vi "phil_visualize.vi"() -> ()   [LabVIEW 2016]
uses:
  <userlib>/LevyLab/Graph Utilities/Typedefs/Histogram--slider.ctl
  subvi/ctl/Scan Info -- Cluster.ctl
  subvi/ctl/Chopper Parameters -- Cluster.ctl
  <userlib>/LevyLab/Graph Utilities/Typedefs/Histogram--Graph.ctl
  <userlib>/LevyLab/Graph Utilities/graph_utilities.lvclass
  <userlib>/LevyLab/LV to ITX/Data/Data.lvclass
  subvi/Data.S3/Data.S3.lvclass
  <userlib>/LevyLab/postgreSQL-timescaleDB/Data.PGSQL.lvclass
  <userlib>/LevyLab/Graph Utilities/graph_utilities.lvclass/graph_utilities.ctl
  <userlib>/LevyLab/LV to ITX/Data/Data.lvclass/Data.ctl
  subvi/operationQueue/fft/fft_typedef.ctl
  subvi/operationQueue/derivative/derivative_typedef.ctl
  <userlib>/_OpenG.lib/file/file.llb/File Exists - Scalar__ogtk.vi
  <userlib>/_OpenG.lib/file/file.llb/Build Path - Traditional__ogtk.vi
  <userlib>/_OpenG.lib/file/file.llb/Strip Path - Traditional__ogtk.vi
  <userlib>/_OpenG.lib/dictionary/dictionary.llb/Dictionary Update (by scalar value)__ogtk.vi
  <userlib>/LevyLab/XY Utilities/subVIs/Derivative (multiple).vi
  <userlib>/LevyLab/XY Utilities/xy_utilities.lvlib
panel:
  in  "Tab Control":enum32{"Graphs", "Page 2"}(tab)
  out "Horizontal Linecut":cluster{dbl[], dbl[]}[](graph)
  out "Vertical Linecut":cluster{dbl[], dbl[]}[](graph)
  out "Intensity Graph":dbl[][](graph)
  out "Histogram":T1
  in  "lock to bin edges":bool
  in  "# std deviations for histogram width":T2=1.4340101522842639 scale=0.0..5.0
  in  "menu select":T3(tab)
  out "Listing Indicator":bool
  out "Downloading Indicator":bool
  in  "Populate Local Tree":bool
  in  "Local Tree":string(tree)
  in  "Populate Remote Tree":bool
  in  "local bigdata directory":path=path "C:/visualization" caption="Path"
  out "Loading Indicator":bool
  out "TDMS load (ms)":u32
  in  "Remote Tree":string(tree)
  in  "path to aws credentials":path=path "C:/Users/patrick/.aws/credentials"
  in  "S3 bucket":string="levylab-data"
  out "Remote Tree load (ms)":u32
  in  "Operation Config":enum32{"derivative", "fft"}(tab)
  in  "derivative":T4={"derivative"="derivative", "Interval"=2.0, "Interval Units"=enum."Points", "Type"=enum."dy/dx vs x"}
  in  "Add Op":bool
  in  "Operations List":i32(listbox)
  in  "update":bool
  out "slicing\ntime":i32
  out "updating":bool
  in  "auto\nupdate":bool
  in  "trash can":i32(listbox)
  in  "'Z' Scale Selection (IV Y)":string(tree)
  in  "'Y' Scale Selection (IV X)":string(tree)
  out "intended sweep end":dbl
  out "actual sweep end":dbl
  in  "intended (t) end\nactual (f) end":bool
  out "scan info":T5
  in  "chopper params":T6
  out "data dimensions":i32[](array[numeric])
  out "wiring config":string[][](array[string])
  out "Notes":string
  out "Wavenames":string[](array[string])
  # "don't try to open a file that's\ncurrently downloading.."
  # "#todo: change these indicator booleans to string-based \"status\" or enum"
  # "not yet implemented"
  # "no settings"
  # "FACTS"
  # "you may find that AI7 and AI8 were not saved\ndue to an old bug in the transport stuff a while ago..\nvery unfortunate"
  # "this does virtually nothing and i am rly confused"
  # "temporary things:"
  # "Settings"
  # "4"
  # "7"
  # "10"
  # "12"
  # "14"
  # "TODO: \n-multiple file download\n-download progress indicator\n-read metadata from tdms"
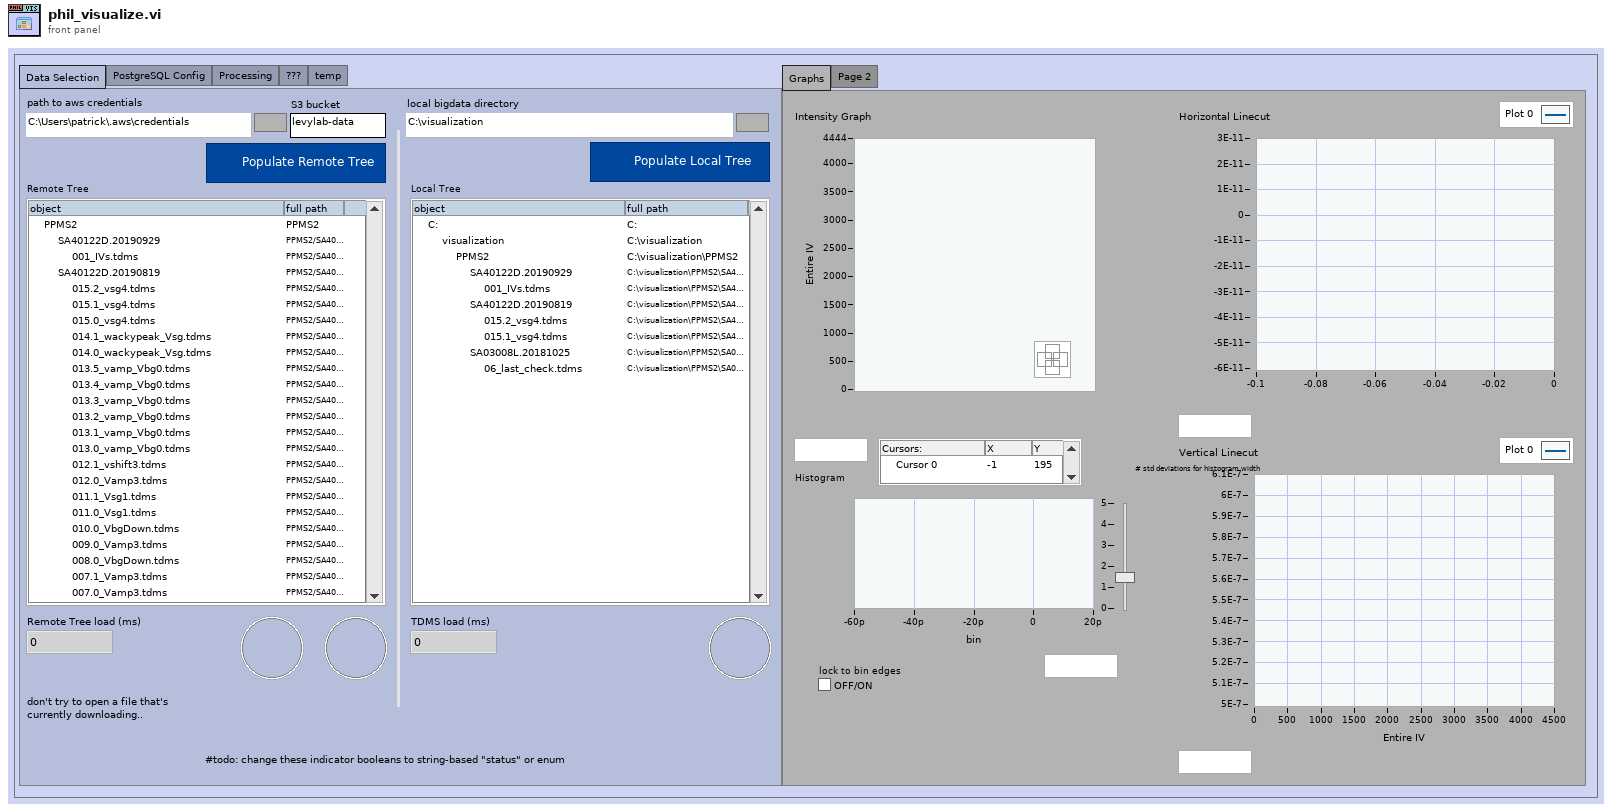
[diagram p1: front panel]
types:
  T1 = typedef "graph_utilities.lvclass/Histogram--Graph.ctl" = cluster{"X":dbl, "Y":dbl}[]
  T2 = typedef "graph_utilities.lvclass/Histogram--slider.ctl" = dbl
  T3 = enum32{"Data Selection", "PostgreSQL Config", "Processing", "???", "temp"}
  T4 = cluster{"derivative":string, "Interval":dbl, "Interval Units":enum16{"Points", "Data"}, "Type":enum16{"dy/dx vs x", "dx/dy vs y"}}
  T5 = typedef "Scan Info -- Cluster.ctl" = cluster{"scan names":string[], "starts":dbl[], "ends":dbl[], "steps":dbl[]}
  T6 = typedef "Chopper Parameters -- Cluster.ctl" = cluster{"Points to chop off the top edge":i32, "Points to chop off the bottom edge":i32, "zeroes to chop off":i32, "use auto-chopper":bool, "upper (t) or lower (f) side":bool}
  T7 = enum32{"Invalid", "Standard", "Closed", "Hidden", "Minimized", "Maximized"}
  T8 = enum32{"invalid app kind", "Development System", "Run Time System", "Student Edition", "Embedded LabVIEW", "Evaluation", "Custom"}
  T9 = typedef "fft_typedef.ctl" = cluster{"fft":string}
  T10 = typedef "derivative_typedef.ctl" = cluster{"derivative":string, "Interval":dbl, "Interval Units":enum16{"Points", "Data"}, "Type":enum16{"dy/dx vs x", "dx/dy vs y"}}
  T11 = typedef "Dictionary Object RefNum__ogtk.ctl" = refnum<k1>
  T12 = cluster{"Core":cluster{"Current VI Reference":refnum<vi>, "Close Panel on Exit?":bool}, "active XY data":cluster{"All expt data":dbl[], "All expt data":dbl[]}[], "local bigdata directory":path, "Data Save":refnum<class "Data.lvclass">, "Data.S3":refnum<class "Data.S3.lvclass">, "Data.PGSQL":refnum<class "Data.PGSQL.lvclass">, "graphs":refnum<class "graph_utilities.lvclass">[], "dictionary out":T11, "Operations List":refnum<vi>, "operations performed":string[], "Histogram Data":cluster{"X Values":dbl[], "Histogram: h(x)":i32[]}, "wavenames":string[], "data dimensions":i32[], "selected":cluster{"local path":path, "\\ remote path":string, "/ remote path":string}, "scan info":cluster{"scan names":string[], "starts":dbl[], "ends":dbl[], "steps":dbl[]}, "wiring config":string[][], "channel selection trees":cluster{"X Scale Selection":refnum<vi>, "Y Scale Selection":refnum<vi>}, "ch selection":cluster{"X Ch":string, "Y Ch":string}}
  T13 = cluster{"X Scale Selection":refnum<vi>, "Y Scale Selection":refnum<vi>}
  T14 = cluster{"scan names":string[], "starts":dbl[], "ends":dbl[], "steps":dbl[]}
  T15 = cluster{"local path":path, "\\ remote path":string, "/ remote path":string}
  T16 = cluster{"X Values":dbl[], "Histogram: h(x)":i32[]}
  T17 = cluster{"All expt data":dbl[], "All expt data":dbl[]}[]
  T18 = cluster{"Current VI Reference":refnum<vi>, "Close Panel on Exit?":bool}
  T19 = typedef "Data.lvclass/Dictionary--cluster.ctl" = cluster{"key":string, "value":variant}
  T20 = cluster{"concatenated string":string, "derivative":cluster{"derivative":string, "Interval":dbl, "Interval Units":enum16{"Points", "Data"}, "Type":enum16{"dy/dx vs x", "dx/dy vs y"}}}
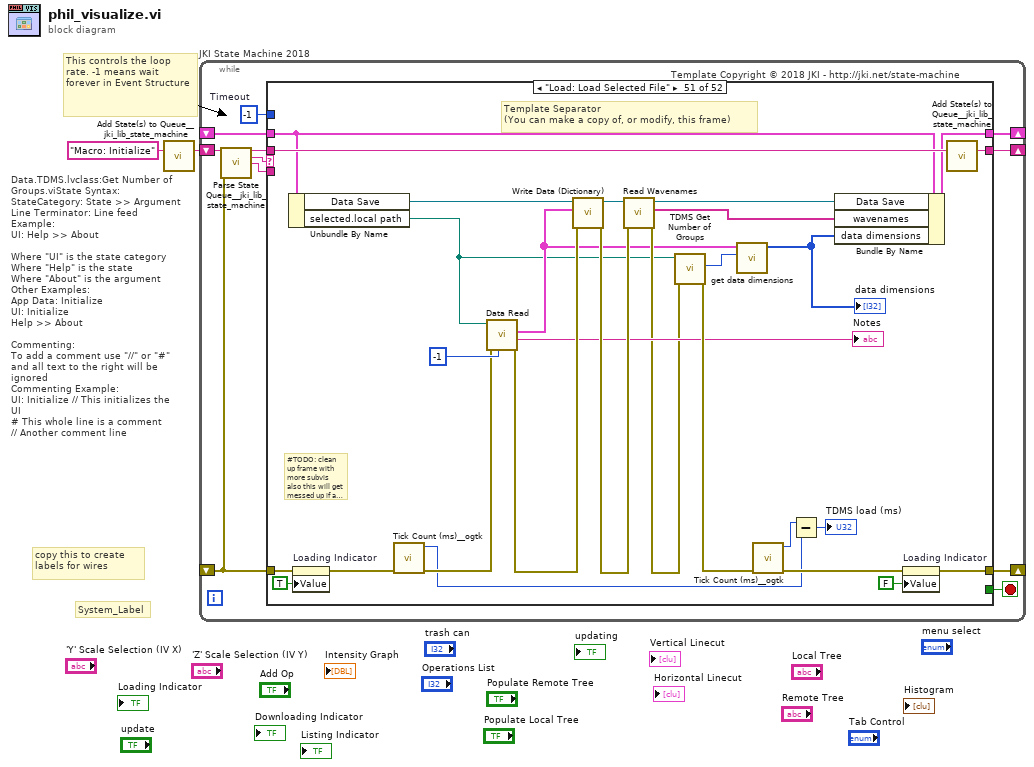
[diagram p0: block diagram]
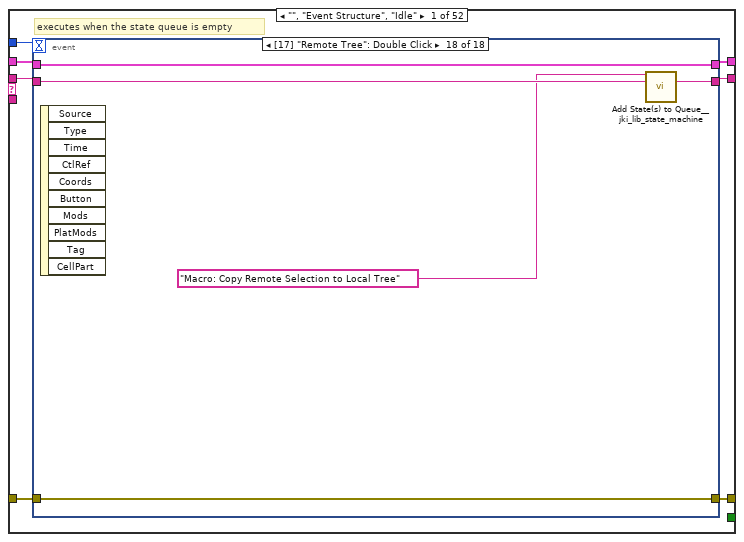
[diagram p2: hidden frame]
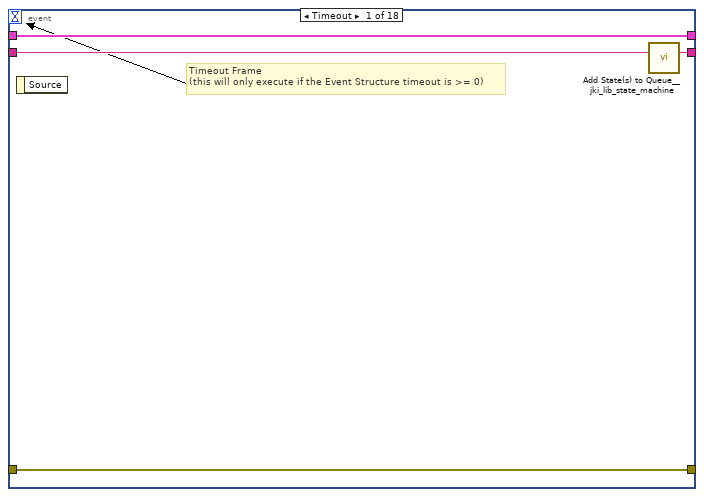
[diagram p3: hidden frame]
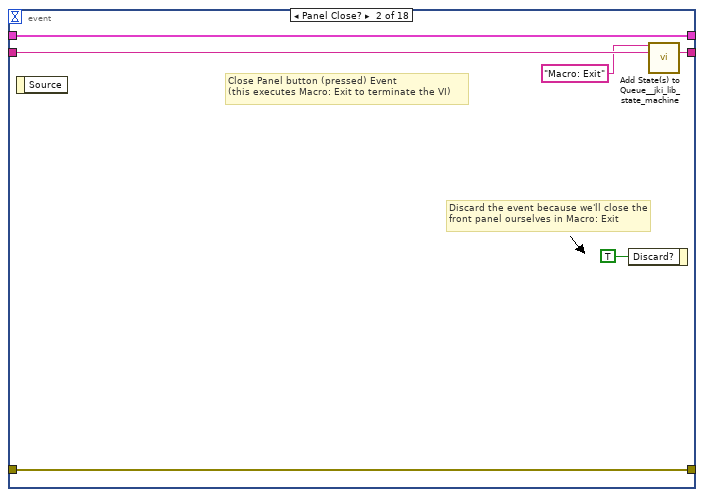
[diagram p4: hidden frame]
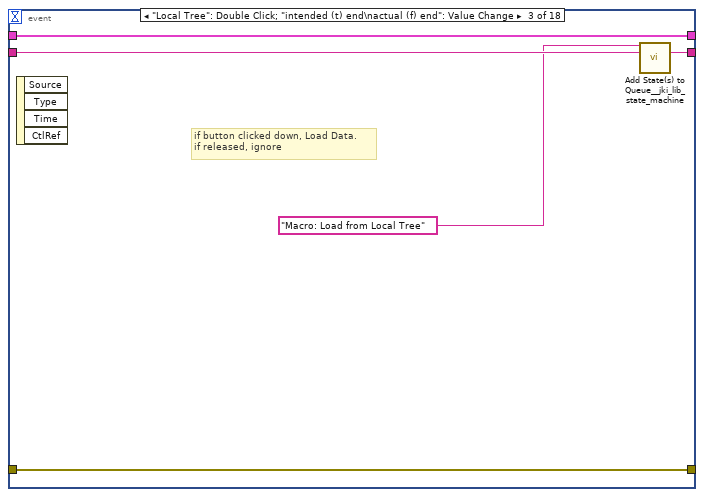
[diagram p5: hidden frame]
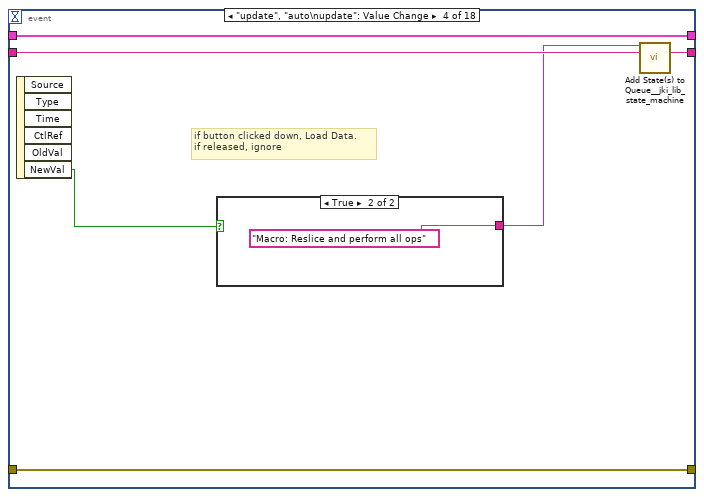
[diagram p6: hidden frame]
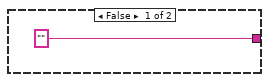
[diagram p7: hidden frame]
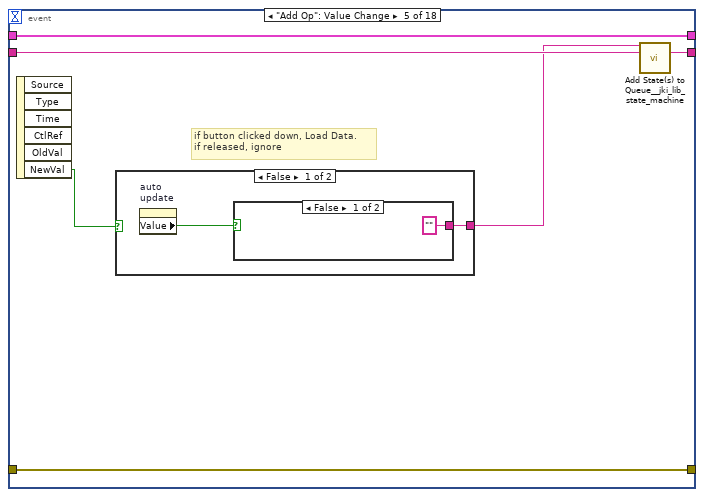
[diagram p8: hidden frame]
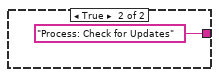
[diagram p9: hidden frame]
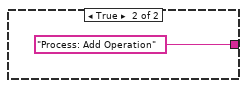
[diagram p10: hidden frame]
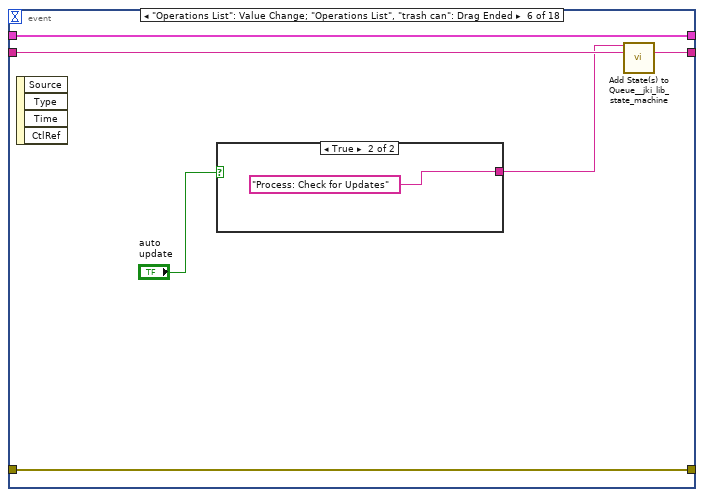
[diagram p11: hidden frame]
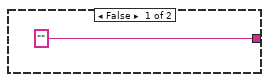
[diagram p12: hidden frame]
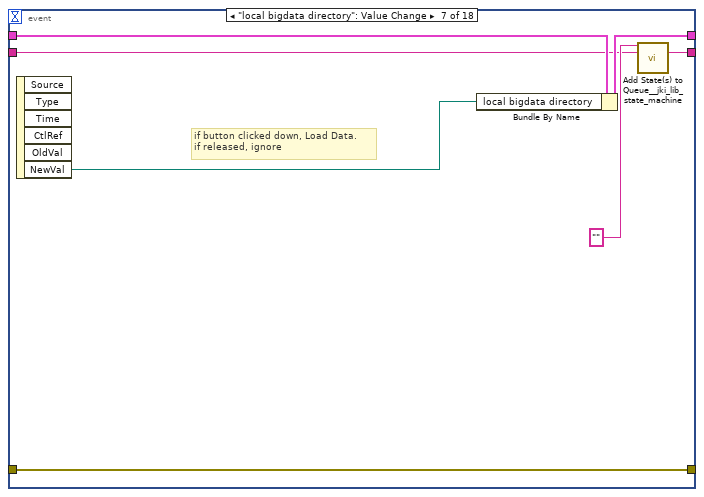
[diagram p13: hidden frame]
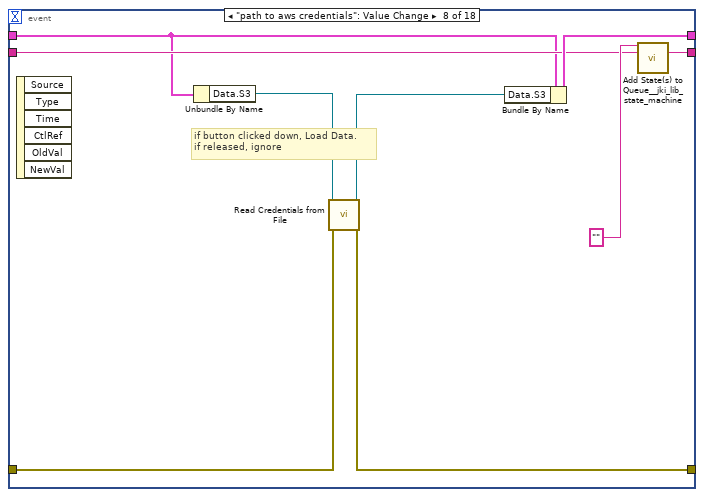
[diagram p14: hidden frame]
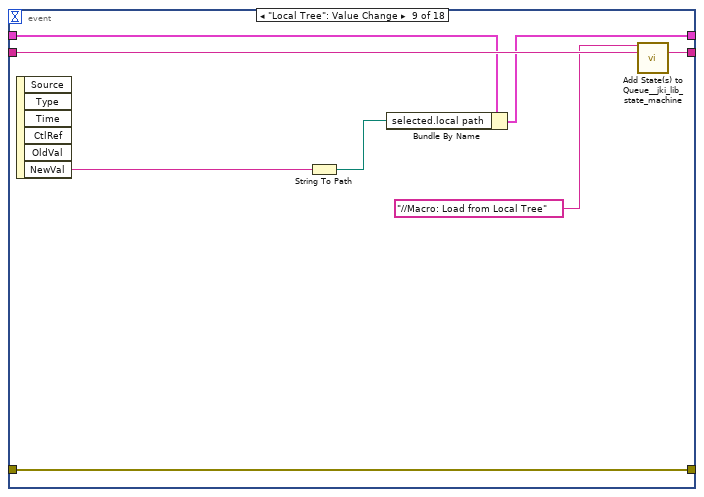
[diagram p15: hidden frame]
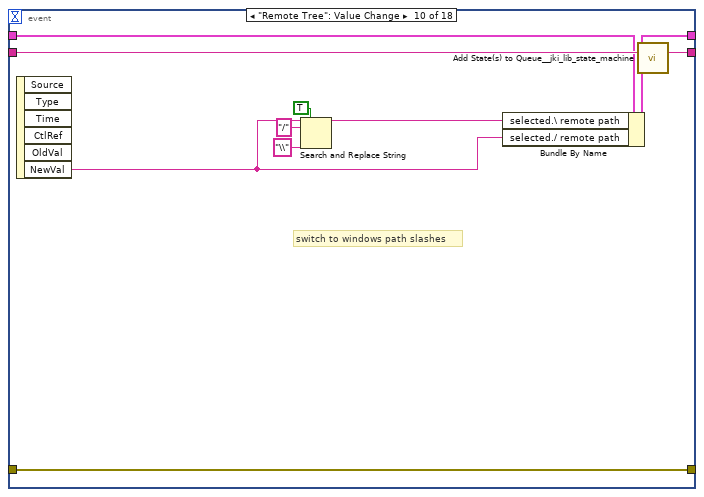
[diagram p16: hidden frame]
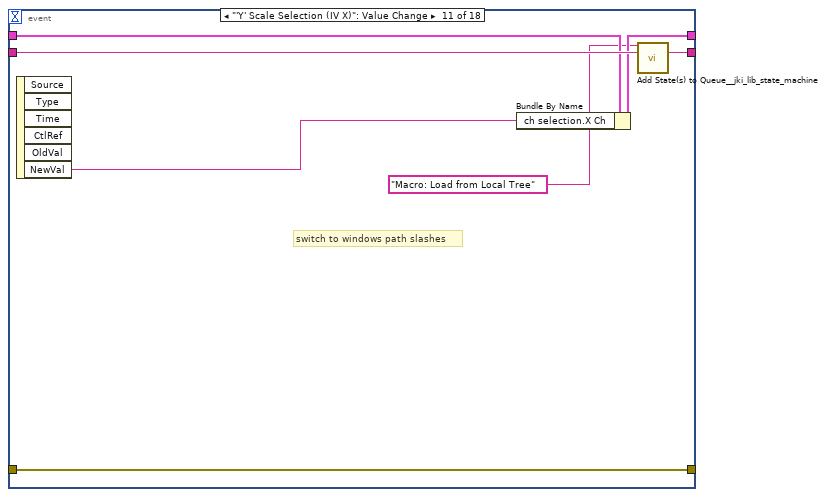
[diagram p17: hidden frame]
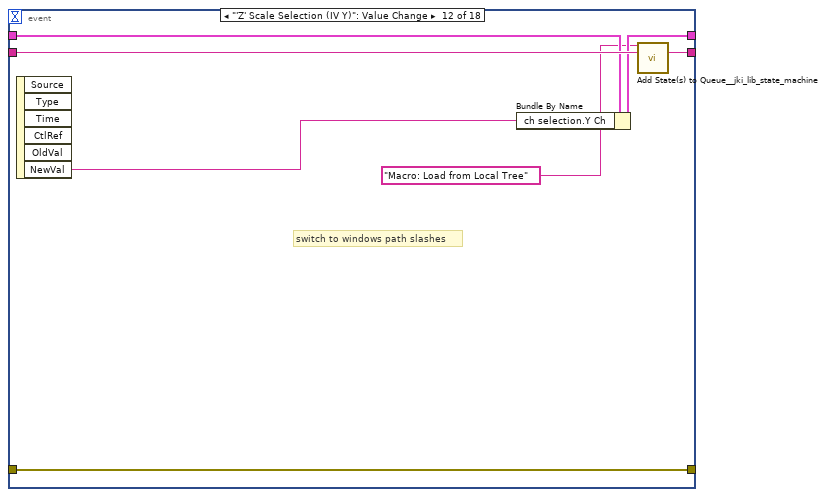
[diagram p18: hidden frame]
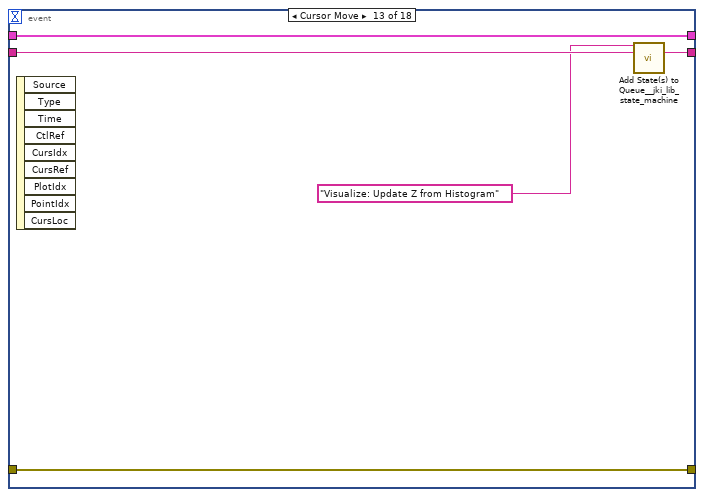
[diagram p19: hidden frame]
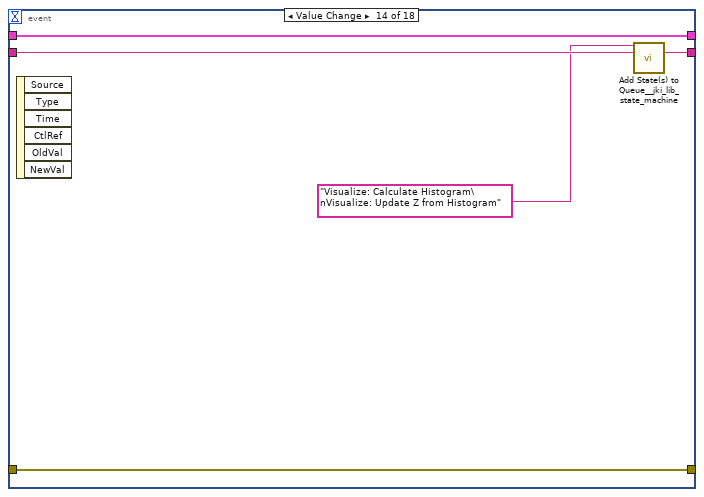
[diagram p20: hidden frame]
diagram:
  # "Data.TDMS.lvclass:Get Number of Groups.viState Syntax:\nStateCategory: State >> Argument\nLine Terminator: Line feed\nExample:\nUI: Help >> About\n\nWhere \"UI\" is the state category\nWhere \"Help\" is the state\nWhere \"About\" is the argument\nOther Examples:\nApp Data: Initialize\nUI: Initialize\nHelp >> About\n\nCommenting:\nTo add a comment use \"//\" or \"#\" and all text to the right will be ignored\nCommenting Example:\nUI: Initialize // This initializes the UI\n# This whole line is a comment\n// Another comment line"
  # "copy this to create labels for wires"
  # "This controls the loop rate. -1 means wait forever in Event Structure"
  # "System_Label"
  n1 = call <vilib>:"Add State(s) to Queue__jki_lib_state_machine.vi"("State(s) in (\"\")"="Macro: Initialize") -> ("States Out"=w2:string)  [unwired: 14 in]
  n2 = while "JKI State Machine 2018" {
    shift-right: [w6] -> _
    shift-left: _ -> [w3]
    shift-right: [w9] -> _
    shift-left: _ -> [w4]
    shift-right: [w8] -> _
    shift-left: w2 -> [w10]
    stop <- w7 stop-if-true
    w5 = -1  # Timeout
    # "Template Copyright © 2018 JKI - http://jki.net/state-machine"
    n3 = call <vilib>:"Parse State Queue__jki_lib_state_machine.vi"("State Queue"=w10, "Error In (no error)"=w4) -> ("Remaining States"=w12:string, "Current State"=w13:string, "Arguments"=w11:string)  [unwired: 11 in]
    n4 = case shown="\"Load: Load Selected File\"" w13 {
      selector: w13 -> [_ _ w151 _ _ _ _ _ _ _ _ _ _ _ _ _ _ _ _ _ _ _ _ _ _ _ _ _ _ _ _ _ _ _ _ _ _ _ _ _ _ _ _ _ _ _ _ _ _ _ _ _]
      tunnel: w12 -> [w20 w150 w155 w174 w175 w185 w189 w217 w239 w245 w249 w258 w264 w275 w344 w349 w359 w366 w371 w376 w381 w386 w391 w396 w406 w410 w414 w418 w422 w434 w452 w473 w496 w517 w529 w533 w541 w545 w549 w569 w589 w594 w620 w657 w703 w712 w732 w774 w778 w791 w823 w839]
      tunnel: w11 -> [_ _ _ _ _ _ _ _ _ _ _ _ w259 w269 _ _ _ _ _ _ _ _ _ _ _ _ _ _ _ _ _ _ _ _ _ _ _ _ _ _ _ _ _ _ _ _ _ _ _ _ _ _]
      tunnel: w3 -> [w18 w147 w153 w167 w178 w183 w186 _ w230 w240 w246 w256 w262 w271 w341 w346 w355 w363 w368 w373 w378 w383 w388 w393 w403 w407 w411 w415 w419 w430 w448 w467 w481 w505 w527 w530 w534 w542 w546 w571 w590 w600 w623 w654 w658 w708 w730 w765 w775 w789 w817 w837]
      tunnel: [w17 w148 w157 w171 errorcluster {"status"=FALSE, "code"=0, "source"=""} ("error out") w182 w187 w212 w235 w241 w247 w254 w260 w272 w342 w347 w356 w362 w367 w372 w377 w382 w387 w392 w404 w408 w412 w416 w420 w423 w435 w458 w489 w513 w523 w531 w537 w543 w547 w574 w592 w602 w624 w655 w697 w709 w728 w766 w776 w787 w819 w826] -> w9
      tunnel: w4 -> [w16 w148 w156 w171 w177 w182 w187 w213 w227 w242 w247 w255 w261 w273 w342 w347 w356 w362 w367 w372 w377 w382 w387 w392 w404 w408 w412 w416 w420 w424 w440 w462 w484 w510 w524 w531 w538 w543 w547 w575 w592 w603 w624 w655 w678 w710 w729 w767 w776 w783 w821 w835]
      tunnel: [w19 w149 w154 w173 w180 w184 w188 w216 w238 w244 w248 w257 w263 w274 w343 w348 w358 w365 w370 w375 w380 w385 w390 w395 w405 w409 w413 w417 w421 w433 w451 w472 w495 w516 w528 w532 w540 w544 w548 w569 w588 w594 w620 w656 w702 w711 w731 w773 w777 w790 w822 w838] -> w8
      tunnel: [_ _ _ _ _ TRUE _ _ _ _ _ _ _ _ _ _ _ _ _ _ _ _ _ _ _ _ _ _ _ _ _ _ _ _ _ _ _ _ _ _ _ _ _ _ _ _ _ _ _ _ _ _] -> w7
      tunnel: [w15 w147 w153 w172 w178 w183 w186 w195 w237 w240 w246 w256 w262 w271 w341 w346 w355 w363 w368 w373 w378 w383 w388 w393 w403 w407 w411 w415 w419 w429 w446 w466 w479 w505 w527 w530 w536 w542 w546 w570 w590 w600 w622 w654 w658 w708 w730 w765 w775 w789 w816 w836] -> w6
      tunnel: w5 -> [w14 _ _ _ _ _ _ _ _ _ _ _ _ _ _ _ _ _ _ _ _ _ _ _ _ _ _ _ _ _ _ _ _ _ _ _ _ _ _ _ _ _ _ _ _ _ _ _ _ _ _ _]
      frame "", "Event Structure", "Idle" {
        # "executes when the state queue is empty"
        n5 = event shown="[17] \"Remote Tree\": Double Click" {
          selector: _ -> [_ _ _ _ _ _ _ _ _ _ _ _ _ _ _ _ _ _]
          dyn-events: _ -> [_ _ _ _ _ _ _ _ _ _ _ _ _ _ _ _ _ _]
          timeout: w14 -> [_ _ _ _ _ _ _ _ _ _ _ _ _ _ _ _ _ _]
          tunnel: w20 -> [w24 w30 w32 w38 w46 w59 w64 w75 w84 w94 w101 w108 w113 w118 w122 w130 w138 w143]
          tunnel: [w23 w29 w33 w39 w47 w58 w65 w76 w85 w95 w102 w109 w112 w117 w123 w131 w139 w144] -> w19
          tunnel: w18 -> [w21 w27 w35 w41 w49 w55 w68 w74 w83 w93 w100 w107 w115 w120 w125 w133 w141 w146]
          tunnel: [w22 w28 w34 w40 w48 w60 w69 w70 w86 w96 w103 w110 w114 w119 w124 w132 w140 w145] -> w17
          tunnel: w16 -> [w22 w28 w34 w40 w48 w60 w69 w71 w86 w96 w103 w110 w114 w119 w124 w132 w140 w145]
          tunnel: [w21 w27 w35 w41 w49 w55 w67 w78 w82 w92 w99 w106 w115 w120 w125 w133 w141 w146] -> w15
          event Timeout {
            # "Timeout Frame\n(this will only execute if the Event Structure timeout is >= 0)"
            n6 = event-data() -> ()  [unwired: 1 in, 1 out]
            n7 = call <vilib>:"Add State(s) to Queue__jki_lib_state_machine.vi"("State(s) in (\"\")"=w24) -> ("States Out"=w23:string)  [unwired: 14 in]
          }
          event Panel Close? {
            # "Discard the event because we'll close the front panel ourselves in Macro: Exit"
            # "Close Panel button (pressed) Event\n(this executes Macro: Exit to terminate the VI)"
            n8 = event-data() -> ()  [unwired: 1 in, 1 out]
            n9 = event-data("Discard?"=TRUE) -> ()  [unwired: 1 in, 1 out]
            n10 = call <vilib>:"Add State(s) to Queue__jki_lib_state_machine.vi"("State(s) in Front (\"\")"="Macro: Exit", "State(s) in (\"\")"=w30) -> ("States Out"=w29:string)  [unwired: 13 in]
          }
          event "Local Tree": Double Click; "intended (t) end\nactual (f) end": Value Change {
            # "if button clicked down, Load Data.\nif released, ignore"
            n11 = event-data() -> ()  [unwired: 1 in, 4 out]
            n12 = call <vilib>:"Add State(s) to Queue__jki_lib_state_machine.vi"("State(s) in Front (\"\")"="Macro: Load from Local Tree", "State(s) in (\"\")"=w32) -> ("States Out"=w33:string)  [unwired: 13 in]
          }
          event "update", "auto\nupdate": Value Change {
            # "if button clicked down, Load Data.\nif released, ignore"
            n13 = event-data() -> ("NewVal"=w37:bool)  [unwired: 1 in, 5 out]
            n14 = case shown="True" w37 {
              tunnel: ["" "Macro: Reslice and perform all ops"] -> w36
              frame False {
              }
              frame True {
              }
            }
            n15 = call <vilib>:"Add State(s) to Queue__jki_lib_state_machine.vi"("State(s) in Front (\"\")"=w36, "State(s) in (\"\")"=w38) -> ("States Out"=w39:string)  [unwired: 13 in]
          }
          event "Add Op": Value Change {
            # "if button clicked down, Load Data.\nif released, ignore"
            n16 = event-data() -> ("NewVal"=w45:bool)  [unwired: 1 in, 5 out]
            n17 = case shown="False" w45 {
              tunnel: [w51 "Process: Add Operation"] -> w44
              frame False {
                n18 = property on="auto\nupdate" class="Bool (strict)"() -> ("Value"=w50:bool)  [unwired: 2 in, 2 out]
                n19 = case shown="False" w50 {
                  tunnel: ["" "Process: Check for Updates"] -> w51
                  frame False {
                  }
                  frame True {
                  }
                }
              }
              frame True {
              }
            }
            n20 = call <vilib>:"Add State(s) to Queue__jki_lib_state_machine.vi"("State(s) in Front (\"\")"=w44, "State(s) in (\"\")"=w46) -> ("States Out"=w47:string)  [unwired: 13 in]
          }
          event "Operations List": Value Change; "Operations List", "trash can": Drag Ended {
            n21 = event-data() -> ()  [unwired: 1 in, 4 out]
            n22 = case shown="True" "auto\nupdate" {
              tunnel: ["" "Process: Check for Updates"] -> w57
              frame False {
              }
              frame True {
              }
            }
            n23 = call <vilib>:"Add State(s) to Queue__jki_lib_state_machine.vi"("State(s) in Front (\"\")"=w57, "State(s) in (\"\")"=w59) -> ("States Out"=w58:string)  [unwired: 13 in]
          }
          event "local bigdata directory": Value Change {
            # "if button clicked down, Load Data.\nif released, ignore"
            n24 = event-data() -> ("NewVal"=w63:path)  [unwired: 1 in, 5 out]
            n25 = Bundle By Name(cluster=w68, "local bigdata directory"=w63) -> (w67:T12)
            n26 = call <vilib>:"Add State(s) to Queue__jki_lib_state_machine.vi"("State(s) in Front (\"\")"="" ("State(s) in Front (\"\")"), "State(s) in (\"\")"=w64) -> ("States Out"=w65:string)  [unwired: 13 in]
          }
          event "path to aws credentials": Value Change {
            # "if button clicked down, Load Data.\nif released, ignore"
            n27 = event-data() -> ()  [unwired: 1 in, 6 out]
            n28 = Unbundle By Name(w74) -> ("Data.S3"=w73:refnum<class "Data.S3.lvclass">)
            n29 = call "Read Credentials from File.vi"("error in (no error)"=w71, "Data.S3"=w73) -> ("error out"=w70:errorcluster, "Data.S3 out"=w72:refnum<class "Data.S3.lvclass">)  [unwired: 8 in]
            n30 = Bundle By Name(cluster=w74, "Data.S3"=w72) -> (w78:T12)
            n31 = call <vilib>:"Add State(s) to Queue__jki_lib_state_machine.vi"("State(s) in Front (\"\")"="" ("State(s) in Front (\"\")"), "State(s) in (\"\")"=w75) -> ("States Out"=w76:string)  [unwired: 13 in]
          }
          event "Local Tree": Value Change {
            n32 = event-data() -> ("NewVal"=w80:string)  [unwired: 1 in, 5 out]
            n33 = String To Path(string=w80) -> (path=w81:path)
            n34 = Bundle By Name(cluster=w83, "selected.local path"=w81) -> (w82:T12)
            n35 = call <vilib>:"Add State(s) to Queue__jki_lib_state_machine.vi"("State(s) in Front (\"\")"="//Macro: Load from Local Tree", "State(s) in (\"\")"=w84) -> ("States Out"=w85:string)  [unwired: 13 in]
          }
          event "Remote Tree": Value Change {
            # "switch to windows path slashes"
            n36 = event-data() -> ("NewVal"=w88:string)  [unwired: 1 in, 5 out]
            n37 = Search and Replace String(replace all?=TRUE ("replace all? (F)"), input string=w88, search string="/", replace string="\\" ("replace string (\"\")")) -> (result string=w89:string)  [unwired: 4 in, 3 out]
            n38 = Bundle By Name(cluster=w93, "selected.\\ remote path"=w89, "selected./ remote path"=w88) -> (w92:T12)
            n39 = call <vilib>:"Add State(s) to Queue__jki_lib_state_machine.vi"("State(s) in (\"\")"=w94) -> ("States Out"=w95:string)  [unwired: 14 in]
          }
          event "'Y' Scale Selection (IV X)": Value Change {
            # "switch to windows path slashes"
            n40 = event-data() -> ("NewVal"=w98:string)  [unwired: 1 in, 5 out]
            n41 = Bundle By Name(cluster=w100, "ch selection.X Ch"=w98) -> (w99:T12)
            n42 = call <vilib>:"Add State(s) to Queue__jki_lib_state_machine.vi"("State(s) in Front (\"\")"="Macro: Load from Local Tree", "State(s) in (\"\")"=w101) -> ("States Out"=w102:string)  [unwired: 13 in]
          }
          event "'Z' Scale Selection (IV Y)": Value Change {
            # "switch to windows path slashes"
            n43 = event-data() -> ("NewVal"=w105:string)  [unwired: 1 in, 5 out]
            n44 = Bundle By Name(cluster=w107, "ch selection.Y Ch"=w105) -> (w106:T12)
            n45 = call <vilib>:"Add State(s) to Queue__jki_lib_state_machine.vi"("State(s) in Front (\"\")"="Macro: Load from Local Tree", "State(s) in (\"\")"=w108) -> ("States Out"=w109:string)  [unwired: 13 in]
          }
          event Cursor Move {
            n46 = event-data() -> ()  [unwired: 1 in, 9 out]
            n47 = call <vilib>:"Add State(s) to Queue__jki_lib_state_machine.vi"("State(s) in Front (\"\")"="Visualize: Update Z from Histogram" ("State(s) in Front (\"\")"), "State(s) in (\"\")"=w113) -> ("States Out"=w112:string)  [unwired: 13 in]
          }
          event Value Change {
            n48 = event-data() -> ()  [unwired: 1 in, 6 out]
            n49 = call <vilib>:"Add State(s) to Queue__jki_lib_state_machine.vi"("State(s) in Front (\"\")"="Visualize: Calculate Histogram\nVisualize: Update Z from Histogram" ("State(s) in Front (\"\")"), "State(s) in (\"\")"=w118) -> ("States Out"=w117:string)  [unwired: 13 in]
          }
          event "Intensity Graph": Cursor Move {
            n50 = event-data() -> ()  [unwired: 1 in, 9 out]
            n51 = call <vilib>:"Add State(s) to Queue__jki_lib_state_machine.vi"("State(s) in Front (\"\")"="Visualize: Line Cuts" ("State(s) in Front (\"\")"), "State(s) in (\"\")"=w122) -> ("States Out"=w123:string)  [unwired: 13 in]
          }
          event "Populate Remote Tree": Value Change {
            n52 = event-data() -> ("NewVal"=w129:bool)  [unwired: 1 in, 5 out]
            n53 = Select(t="Macro: Populate Remote Tree" ("State(s) in Front (\"\")"), s=w129, f="") -> (s? t:f=w126:string)
            n54 = call <vilib>:"Add State(s) to Queue__jki_lib_state_machine.vi"("State(s) in Front (\"\")"=w126, "State(s) in (\"\")"=w130) -> ("States Out"=w131:string)  [unwired: 13 in]
          }
          event "Populate Local Tree": Value Change {
            n55 = event-data() -> ("NewVal"=w137:bool)  [unwired: 1 in, 5 out]
            n56 = Select(t="Macro: Populate Local Tree" ("State(s) in Front (\"\")"), s=w137, f="") -> (s? t:f=w134:string)
            n57 = call <vilib>:"Add State(s) to Queue__jki_lib_state_machine.vi"("State(s) in Front (\"\")"=w134, "State(s) in (\"\")"=w138) -> ("States Out"=w139:string)  [unwired: 13 in]
          }
          event "Remote Tree": Double Click {
            n58 = event-data() -> ()  [unwired: 1 in, 10 out]
            n59 = call <vilib>:"Add State(s) to Queue__jki_lib_state_machine.vi"("State(s) in Front (\"\")"="Macro: Copy Remote Selection to Local Tree" ("State(s) in Front (\"\")"), "State(s) in (\"\")"=w143) -> ("States Out"=w144:string)  [unwired: 13 in]
          }
        }
      }
      frame "---------- Core ----------" {
        # "Do not put any code in this frame.\n(it is a separator no-op)"
        n60 = call <vilib>:"Add State(s) to Queue__jki_lib_state_machine.vi"("State(s) in (\"\")"=w150) -> ("States Out"=w149:string)  [unwired: 14 in]
      }
      frame Default {
        w160 = 42 items=["No error", "Argument error", "Memory is full", "Out of zone", "End of file", "File already open", "Generic file I/O error", "File not found", "File permission error", "Disk is full", "Duplicate path", "Too many files open", "System feature not enabled", "Resource file not found", "Cannot add resource", "Resource not found", "Image not found", "Image memory error", "Pen does not exist", "Config type invalid", "Config token not found", "Config parse error", "Config memory error", "Bad external code format", "Bad external code offset", "External code not present", "Null window", "Destroy window error", "Null menu", "Print aborted", "Bad print record", "Print driver error", "Windows error during printing", "Memory error during printing", "Print dialog error", "Generic print error", "Invalid device refnum", "Device not found", "Device parameter error", "Device unit error", "Cannot open device", "Device call aborted", "Generic error", "Cancelled by user", "Object ID too low", "Object ID too high", "Object not in heap", "Unknown heap", "Unknown object (invalid DefProc)", "Unknown object (DefProc not in table)", "Message out of range", "Invalid (null) method", "Unknown message", "Manager call not supported", "Bad address", "Network operation in progress", "Network operation timed out", "Connection is busy", "Network attribute not supported", "Network error", "Address in use", "System out of memory", "Connection aborted", "Connection refused", "Not connected", "Already connected", "Connection closed", "Initialization error (interapplication manager)", "Bad occurrence", "Wait on unbound occurrence handler", "Occurrence queue overflow", "Datalog type conflict", "Unused", "Unrecognized type (interapplication manager)", "Memory corrupt", "Failed to make temporary DLL", "Old CIN version", "Drag socket not found", "Failed to load drop-object", "Failed to register OLE object", "Failed to release OLE object", "Format specifier type mismatch", "Unknown format specifier", "Too few format specifiers", "Too many format specifiers", "Scan failed", "Newer CIN version", "Error converting to variant", "Runtime menu error", "Password tampered", "Variant attribute not found", "Incompatible variant data type", "Event data is not available", "Event Store is not present", "Occurrence is not found", "Event Queue is not created", "Event info is not available", "Refnum passed is NULL", "Error retrieving Class GUID", "Error retrieving CoClass GUID", "Error retrieving TypeLib GUID.", "Bad built application magic bytes.", "Specific driver is different from the specific driver associated with the Logical Name.", "There is no session opened to the class driver.", "Max Error", "MAX - Error with config objects", "MAX - Error loading configuration", "MAX - Group not supported"]
        # "Current State"
        # "Do not delete, rename, or modify this frame.\n(this is used to capture unhandled states and typos)"
        # "Handle mistyped state name (developer tool)"
        n61 = Format Into String(format string="Software Exception: Unhandled State \"%s\"." ("message"), error in=w156, w151) -> (resulting string=w159:string, error out=w158:errorcluster)  [unwired: 1 in]
        n62 = call <vilib>:"Error Cluster From Error Code.vi"("show call chain? (False)"=TRUE, "error in (no error)"=w158, "error message (\"\")"=w159, "error code (0)"=w160) -> ("error out"=w157:errorcluster)  [unwired: 5 in]
        n63 = call <vilib>:"Add State(s) to Queue__jki_lib_state_machine.vi"("State(s) in (\"\")"=w155) -> ("States Out"=w154:string)  [unwired: 14 in]
      }
      frame "Initialize Core Data" {
        # "Do not delete, rename, or modify this frame.\n(this is used to determine panel behavior on exit)"
        # "originally closed?"
        # "exe?"
        # "If panel starts closed or is an EXE, then close it when we exit"
        n64 = property class="VI"() -> ("FP.State"=w164:T7)  [unwired: 2 in, 2 out]
        n65 = property class="App"() -> ("App.Kind"=w170:T8)  [unwired: 2 in, 2 out]
        n66 = control-ref of="Current VI Reference"() -> (w165:refnum<vi>)
        n67 = Equal?(x=w164, y=T7."Closed" ("Front Panel Window:State")) -> (x = y?=w162:bool)
        n68 = Equal?(x=w170, y=T8."Run Time System" ("Application:Kind")) -> (x = y?=w168:bool)
        n69 = Or(x=w162, y=w168) -> (x .or. y?=w166:bool)
        n70 = Bundle By Name(cluster=w167, "Core.Current VI Reference"=w165, "Core.Close Panel on Exit?"=w166) -> (w172:T12)
        n71 = call <vilib>:"Add State(s) to Queue__jki_lib_state_machine.vi"("State(s) in (\"\")"=w174) -> ("States Out"=w173:string)  [unwired: 14 in]
      }
      frame "Error Handler" {
        # "Unhandled Error -- Display it"
        # "Handle any errors here.\nYou can also output any states to clean-up after errors occur"
        # "Clear error"
        n72 = call <vilib>:"General Error Handler.vi"("error in (no error)"=w177) -> ()  [unwired: 10 in, 5 out]
        n73 = call <vilib>:"Add State(s) to Queue__jki_lib_state_machine.vi"("State(s) in Front (\"\")"="/* Post Error States", "State(s) in (\"\")"=w175) -> ("States Out"=w180:string)  [unwired: 13 in]
      }
      frame "Exit" {
        # "Do not put any code in this frame.\n(No errors that occur here will be handled.)"
        n74 = call <vilib>:"Add State(s) to Queue__jki_lib_state_machine.vi"("State(s) in (\"\")"=w185) -> ("States Out"=w184:string)  [unwired: 14 in]
      }
      frame "---------- Data ----------" {
        # "Do not put any code in this frame.\n(It is a separator no-op. You can make a copy of this frame to create a new Data frame)"
        n75 = call <vilib>:"Add State(s) to Queue__jki_lib_state_machine.vi"("State(s) in (\"\")"=w189) -> ("States Out"=w188:string)  [unwired: 14 in]
      }
      frame "Data: Initialize" {
        w191 = refnum<class "Data.PGSQL.lvclass"> refnum  # Data.PGSQL
        w196 = cluster{"X Ch":string, "Y Ch":string} {"X Ch"="AO3", "Y Ch"="AI4"}  # ch selection
        w197 = T13 {"X Scale Selection"=refnum, "Y Scale Selection"=refnum}  # channel selection trees
        w201 = string[][] []  # wiring config
        w202 = T14 {"scan names"=["DSA_Vsg1", "OFF", "OFF", "OFF"], "starts"=[-1.0, 0.0, 0.2, 0.0], "ends"=[1.0, 0.2, 0.3, 0.5], "steps"=[0.005, 0.001, 0.025, 0.01]}  # scan info
        w203 = T15 {"local path"=path "", "\\ remote path"="", "/ remote path"=""}  # selected
        w204 = i32[] []  # data dimensions
        w192 = refnum<class "Data.S3.lvclass"> refnum  # Data.S3
        w205 = string[] []  # wavenames
        w194 = refnum<class "Data.lvclass"> refnum  # Data Save
        w206 = T16 {"X Values"=[], "Histogram: h(x)"=[]}  # Histogram Data
        w207 = string[] []  # operations performed
        w209 = T17 []  # active XY data
        w208 = string[] [] ("Strings []")
        w193 = refnum<class "graph_utilities.lvclass">[] []  # graphs
        w215 = T18 {"Current VI Reference"=refnum, "Close Panel on Exit?"=FALSE}  # Core
        # "# groups in tdms\n    (i.e. # original itx files)\n# channels (time, AIN, AON,\n# points per channel\n    (except the channels\n     that only store 1)"
        # "do not delete - used by framework"
        # "Data names and types of shift register data are defined by this bundle."
        # "Initialize the shift-register data, here.\n(data names are defined by what you wire into the bundle function)"
        n76 = call <userlib>:"Dictionary Create__ogtk.vi"("error in (no error)"=w213) -> ("error out"=w212:errorcluster, "dictionary out"=w214:T11)  [unwired: 9 in]
        n77 = control-ref of="Operations List"() -> (w210:refnum<vi>)
        n78 = property on="trash can" class="LstBox (strict)"("Item Names"=w208) -> ()  [unwired: 2 in, 2 out]
        n79 = property class="LstBox (strict)"(reference=w210, "Item Names"=w208) -> (reference out=w211:refnum<vi>)  [unwired: 1 in, 1 out]
        n80 = control-ref of="'Y' Scale Selection (IV X)"() -> (w200:refnum<vi>)
        n81 = control-ref of="'Z' Scale Selection (IV Y)"() -> (w199:refnum<vi>)
        n82 = Bundle(cluster=w197, "X Scale Selection"=w200, "Y Scale Selection"=w199) -> (w198:T13)
        n83 = Bundle("Core"=w215, "active XY data"=w209, "local bigdata directory"="local bigdata directory", "Data Save"=w194, "Data.S3"=w192, "Data.PGSQL"=w191, "graphs"=w193, "dictionary out"=w214, "Operations List"=w211, "operations performed"=w207, "Histogram Data"=w206, "wavenames"=w205, "data dimensions"=w204, "selected"=w203, "scan info"=w202, "wiring config"=w201, "channel selection trees"=w198, "ch selection"=w196) -> (w195:T12)  [unwired: 1 in]
        n84 = call <vilib>:"Add State(s) to Queue__jki_lib_state_machine.vi"("State(s) in (\"\")"=w217) -> ("States Out"=w216:string)  [unwired: 14 in]
      }
      frame "Data: Initialize Graph References" {
        # "#todo\nmove elsewhere"
        # "clear graph"
        n85 = invoke on="Remote Tree" class="Tree (strict)" method="Edit Tree Items.Delete"(error in=w227) -> (error out=w226:errorcluster)  [unwired: 4 in, 4 out]
        n86 = control-ref of="Intensity Graph"() -> (w218:refnum<vi>)
        n87 = property class="IntGraph (strict)"(reference=w218, "Value"=dbl[][] []) -> (reference out=w228:refnum<vi>)  [unwired: 1 in, 1 out]
        n88 = invoke on="Local Tree" class="Tree (strict)" method="Edit Tree Items.Delete"(error in=w226) -> (error out=w225:errorcluster)  [unwired: 4 in, 4 out]
        n89 = control-ref of="Histogram"() -> (w220:refnum<vi>)
        n90 = control-ref of="Vertical Linecut"() -> (w232:refnum<vi>)
        n91 = control-ref of="Horizontal Linecut"() -> (w233:refnum<vi>)
        n92 = call <userlib>:"Write Intensity Graph ref.vi"("error in (no error)"=w225, "Intensity Graph (Control)"=w228, "Intensity Graph"=w228) -> ("error out"=w222:errorcluster, "graph_utilities out"=w224:refnum<class "graph_utilities.lvclass">)  [unwired: 7 in]
        n93 = call <userlib>:"Write XY Graph ref.vi"("error in (no error)"=w222, "XY Graph"=w220, "graph_utilities in"=w224) -> ("error out"=w221:errorcluster, "graph_utilities out"=w223:refnum<class "graph_utilities.lvclass">)  [unwired: 7 in]
        n94 = call <userlib>:"Write XY Graph ref.vi"("error in (no error)"=w221, "XY Graph"=w232, "graph_utilities in"=w224) -> ("error out"=w236:errorcluster, "graph_utilities out"=w231:refnum<class "graph_utilities.lvclass">)  [unwired: 7 in]
        n95 = call <userlib>:"Write XY Graph ref.vi"("error in (no error)"=w236, "XY Graph"=w233, "graph_utilities in"=w224) -> ("error out"=w235:errorcluster, "graph_utilities out"=w234:refnum<class "graph_utilities.lvclass">)  [unwired: 7 in]
        n96 = Build Array(w223, w231, w234) -> (w219:refnum<class "graph_utilities.lvclass">[])
        n97 = Bundle By Name(cluster=w230, "graphs"=w219) -> (w237:T12)
        n98 = call <vilib>:"Add State(s) to Queue__jki_lib_state_machine.vi"("State(s) in (\"\")"=w239) -> ("States Out"=w238:string)  [unwired: 14 in]
      }
      frame "Data: Cleanup" {
        # "Cleanup any data and references, here.\n(this is called automatically, by the Macro: Exit)"
        n99 = Unbundle By Name(w240) -> ("Core.Current VI Reference"=w243:refnum<vi>)
        n100 = Close Reference(reference=w243, error in (no error)=w242) -> (error out=w241:errorcluster)
        n101 = call <vilib>:"Add State(s) to Queue__jki_lib_state_machine.vi"("State(s) in (\"\")"=w245) -> ("States Out"=w244:string)  [unwired: 14 in]
      }
      frame "---------- UI ----------" {
        # "Do not put any code in this frame.\n(It is a separator no-op. You can make a copy of this frame to create a new UI frame)"
        n102 = call <vilib>:"Add State(s) to Queue__jki_lib_state_machine.vi"("State(s) in (\"\")"=w249) -> ("States Out"=w248:string)  [unwired: 14 in]
      }
      frame "UI: Initialize" {
        w250 = FALSE ("Loading Indicator")
        # "Initialize the User Interface, here.\n(this is called automatically, by the Macro: Init)"
        n103 = call <userlib>:"Fit VI window to Largest Dec__ogtk.vi"("error in (no error)"=w255, "border spacing (2 px)"=-2) -> ("error out"=w254:errorcluster)  [unwired: 4 in, 1 out]
        n104 = local write "Loading Indicator"(w250) -> ()
        n105 = local write "Downloading Indicator"(w250) -> ()
        n106 = local write "Remote Tree load (ms)"(u32 0 ("Remote Tree load (ms)")) -> ()
        n107 = local write "TDMS load (ms)"(u32 0 ("TDMS load (ms)")) -> ()
        n108 = local write "Listing Indicator"(w250) -> ()
        n109 = call <vilib>:"Add State(s) to Queue__jki_lib_state_machine.vi"("State(s) in (\"\")"=w258) -> ("States Out"=w257:string)  [unwired: 14 in]
      }
      frame "UI: Cursor Set" {
        # "Argument"
        # "Set and Unset Cursor Busy.\n(Usage: \"UI: Cursor Set >> Busy|Idle\")"
        n110 = case shown="\"Idle\", Default" w259 {
          tunnel: w261 -> [w266 w268]
          tunnel: [w265 w267] -> w260
          frame "Idle", Default {
            n111 = call <vilib>:"Unset Busy.vi"("error in (no error)"=w266) -> ("error out"=w265:errorcluster)  [unwired: 10 in]
          }
          frame "Busy" {
            n112 = call <vilib>:"Set Busy.vi"("error in (no error)"=w268) -> ("error out"=w267:errorcluster)  [unwired: 9 in, 1 out]
          }
        }
        n113 = call <vilib>:"Add State(s) to Queue__jki_lib_state_machine.vi"("State(s) in (\"\")"=w264) -> ("States Out"=w263:string)  [unwired: 14 in]
      }
      frame "UI: Front Panel State" {
        # "Argument"
        # "Set Front Panel Open or Closed\n(Usage: \"UI: Front Panel State >> Open|Close\")"
        n114 = Unbundle By Name(w271) -> ("Core.Current VI Reference"=w270:refnum<vi>)
        n115 = case shown="\"Minimize\", \"Minimized\"" w269 {
          tunnel: w273 -> [w281 w296 w307 w320 w333]
          tunnel: [w283 w297 w309 w322 w335] -> w272
          tunnel: w270 -> [w282 w294 w308 w321 w334]
          frame "Open", "Standard", Default {
            w276 = T7."Standard" ("State")
            n116 = property class="VI"(reference=w282, error in=w281) -> (reference out=w279:refnum<vi>, error out=w280:errorcluster, "FP.State"=w278:T7)
            n117 = Not Equal?(x=w278, y=w276) -> (x != y?=w277:bool)
            n118 = case shown="True" w277 {
              tunnel: [w287 w289] -> w283
              tunnel: w280 -> [w286 w289]
              tunnel: w279 -> [w285 _]
              tunnel: w276 -> [w284 _]
              frame True {
                n119 = invoke class="VI" method="FP.Open"(reference=w285, error in=w286, "Activate"=TRUE, "State"=w284) -> (error out=w287:errorcluster)  [unwired: 1 in, 4 out]
              }
              frame False {
              }
            }
          }
          frame "Close", "Closed" {
            n120 = property class="VI"(reference=w294, error in=w296) -> (reference out=w293:refnum<vi>, error out=w295:errorcluster, "FP.State"=w291:T7)
            n121 = Not Equal?(x=w291, y=T7."Closed" ("Front Panel Window:State")) -> (x != y?=w290:bool)
            n122 = case shown="True" w290 {
              tunnel: [w298 w301] -> w297
              tunnel: w295 -> [w298 w300]
              tunnel: w293 -> [_ w299]
              frame False {
              }
              frame True {
                n123 = invoke class="VI" method="FP.Close"(reference=w299, error in=w300) -> (error out=w301:errorcluster)  [unwired: 1 in, 2 out]
              }
            }
          }
          frame "Hidden", "Hide" {
            w302 = T7."Hidden" ("State")
            n124 = property class="VI"(reference=w308, error in=w307) -> (reference out=w305:refnum<vi>, error out=w306:errorcluster, "FP.State"=w304:T7)
            n125 = Not Equal?(x=w304, y=w302) -> (x != y?=w303:bool)
            n126 = case shown="True" w303 {
              tunnel: [w313 w314] -> w309
              tunnel: w306 -> [w312 w314]
              tunnel: w305 -> [w311 _]
              tunnel: w302 -> [w310 _]
              frame True {
                n127 = invoke class="VI" method="FP.Open"(reference=w311, error in=w312, "State"=w310) -> (error out=w313:errorcluster)  [unwired: 2 in, 4 out]
              }
              frame False {
              }
            }
          }
          frame "Minimize", "Minimized" {
            w315 = T7."Minimized" ("State")
            n128 = property class="VI"(reference=w321, error in=w320) -> (reference out=w318:refnum<vi>, error out=w319:errorcluster, "FP.State"=w317:T7)
            n129 = Not Equal?(x=w317, y=w315) -> (x != y?=w316:bool)
            n130 = case shown="True" w316 {
              tunnel: [w326 w327] -> w322
              tunnel: w319 -> [w325 w327]
              tunnel: w318 -> [w324 _]
              tunnel: w315 -> [w323 _]
              frame True {
                n131 = invoke class="VI" method="FP.Open"(reference=w324, error in=w325, "State"=w323) -> (error out=w326:errorcluster)  [unwired: 2 in, 4 out]
              }
              frame False {
              }
            }
          }
          frame "Maximize", "Maximized" {
            w328 = T7."Maximized" ("State")
            n132 = property class="VI"(reference=w334, error in=w333) -> (reference out=w331:refnum<vi>, error out=w332:errorcluster, "FP.State"=w330:T7)
            n133 = Not Equal?(x=w330, y=w328) -> (x != y?=w329:bool)
            n134 = case shown="True" w329 {
              tunnel: [w339 w340] -> w335
              tunnel: w332 -> [w338 w340]
              tunnel: w331 -> [w337 _]
              tunnel: w328 -> [w336 _]
              frame True {
                n135 = invoke class="VI" method="FP.Open"(reference=w337, error in=w338, "State"=w336) -> (error out=w339:errorcluster)  [unwired: 2 in, 4 out]
              }
              frame False {
              }
            }
          }
        }
        n136 = call <vilib>:"Add State(s) to Queue__jki_lib_state_machine.vi"("State(s) in (\"\")"=w275) -> ("States Out"=w274:string)  [unwired: 14 in]
      }
      frame "---------- Macro ----------" {
        # "Do not put any code in this frame.\n(It is a separator no-op. You can make a copy of this frame to create a new Macro frame)"
        n137 = call <vilib>:"Add State(s) to Queue__jki_lib_state_machine.vi"("State(s) in (\"\")"=w344) -> ("States Out"=w343:string)  [unwired: 14 in]
      }
      frame "Macro: Initialize" {
        # "Initialization Macro\n(This is called once, when the VI starts)"
        n138 = call <vilib>:"Add State(s) to Queue__jki_lib_state_machine.vi"("State(s) in Front (\"\")"="Data: Initialize\nData: Initialize Graph References\nInitialize Core Data\nUI: Initialize\nUI: Front Panel State >> Open", "State(s) in (\"\")"=w349) -> ("States Out"=w348:string)  [unwired: 13 in]
      }
      frame "Macro: Load from Local Tree" {
        # "Initialization Macro\n(This is called once, when the VI starts)"
        n139 = Unbundle By Name(w355) -> ("selected.local path"=w354:path)
        n140 = call-poly <userlib>:"File Exists__ogtk.vi"("file path"=w354) -> ("is directory"=w353:bool, "exists"=w351:bool)  [unwired: 6 in]
        n141 = Not(x=w353) -> (.not. x?=w352:bool)
        n142 = And(x=w352, y=w351) -> (x .and. y?=w350:bool)
        n143 = case shown="True" w350 {
          tunnel: [" " "UI: Cursor Set >> Busy\nLoad: Load Selected File\nLoad: Load Metadata\nProcess: Slice to XY data\nMacro: Visualize\nUI: Cursor Set >> Idle"] -> w357
          frame False {
            n144 = call "Display Message to User2"() -> ()  [unwired: 10 in, 2 out]
          }
          frame True {
          }
        }
        n145 = call <vilib>:"Add State(s) to Queue__jki_lib_state_machine.vi"("State(s) in Front (\"\")"=w357, "State(s) in (\"\")"=w359) -> ("States Out"=w358:string)  [unwired: 13 in]
      }
      frame "Macro: Populate Remote Tree" {
        # "#TODO: should make sure AWS is configured etc. instead of crashing"
        # "Initialization Macro\n(This is called once, when the VI starts)"
        n146 = call <vilib>:"Add State(s) to Queue__jki_lib_state_machine.vi"("State(s) in Front (\"\")"="UI: Cursor Set >> Busy\nAWS: Initialize\nAWS: Populate Remote Tree\nUI: Cursor Set >> Idle", "State(s) in (\"\")"=w366) -> ("States Out"=w365:string)  [unwired: 13 in]
      }
      frame "Macro: Populate Local Tree" {
        # "#TODO: should make sure path is valid or something"
        # "Initialization Macro\n(This is called once, when the VI starts)"
        n147 = call <vilib>:"Add State(s) to Queue__jki_lib_state_machine.vi"("State(s) in Front (\"\")"="UI: Cursor Set >> Busy\nLoad: Populate Local Tree\nUI: Cursor Set >> Idle", "State(s) in (\"\")"=w371) -> ("States Out"=w370:string)  [unwired: 13 in]
      }
      frame "Macro: Visualize" {
        # "#TODO: should rename this macro,\nit only needs to be sliced after the slicing indices are changed"
        n148 = call <vilib>:"Add State(s) to Queue__jki_lib_state_machine.vi"("State(s) in Front (\"\")"="UI: Cursor Set >> Busy\nVisualize: Plot Live XY to Intensity\nVisualize: Calculate Histogram\nVisualize: Update Z from Histogram\nVisualize: Line Cuts\nUI: Cursor Set >> Idle", "State(s) in (\"\")"=w376) -> ("States Out"=w375:string)  [unwired: 13 in]
      }
      frame "Macro: Upload to AWS" {
        # "#TODO: should rename this macro,\nit only needs to be sliced after the slicing indices are changed"
        # "Initialization Macro\n(This is called once, when the VI starts)"
        n149 = call <vilib>:"Add State(s) to Queue__jki_lib_state_machine.vi"("State(s) in Front (\"\")"="UI: Cursor Set >> Busy\nAWS: Upload file\nUI: Cursor Set >> Idle\n//AWS: Check if file exists", "State(s) in (\"\")"=w381) -> ("States Out"=w380:string)  [unwired: 13 in]
      }
      frame "Macro: Download from AWS" {
        # "#TODO: should rename this macro,\nit only needs to be sliced after the slicing indices are changed"
        # "Initialization Macro\n(This is called once, when the VI starts)"
        n150 = call <vilib>:"Add State(s) to Queue__jki_lib_state_machine.vi"("State(s) in Front (\"\")"="UI: Cursor Set >> Busy\n//AWS: Check if file exists\nAWS: Download file\nUI: Cursor Set >> Idle", "State(s) in (\"\")"=w386) -> ("States Out"=w385:string)  [unwired: 13 in]
      }
      frame "Macro: Copy Remote Selection to Local Tree" {
        # "#TODO: should rename this macro,\nit only needs to be sliced after the slicing indices are changed"
        # "Initialization Macro\n(This is called once, when the VI starts)"
        n151 = call <vilib>:"Add State(s) to Queue__jki_lib_state_machine.vi"("State(s) in Front (\"\")"="UI: Cursor Set >> Busy\nAWS: Copy Remote Selection to Local Tree\nUI: Cursor Set >> Idle", "State(s) in (\"\")"=w391) -> ("States Out"=w390:string)  [unwired: 13 in]
      }
      frame "Macro: Reslice and perform all ops" {
        # "#TODO: should rename this macro,\nit only needs to be sliced after the slicing indices are changed"
        # "Initialization Macro\n(This is called once, when the VI starts)"
        n152 = call <vilib>:"Add State(s) to Queue__jki_lib_state_machine.vi"("State(s) in Front (\"\")"="UI: Cursor Set >> Busy\nProcess: Slice to XY data\nProcess: Perform All Operations\nMacro: Visualize\nUI: Cursor Set >> Idle", "State(s) in (\"\")"=w396) -> ("States Out"=w395:string)  [unwired: 13 in]
      }
      frame "Macro: Exit" {
        # "Exit Macro\n(This is called once, when the VI exits)"
        n153 = Unbundle By Name(w403) -> ("Core.Close Panel on Exit?"=w402:bool)
        n154 = Select(t="UI: Front Panel State >> Close", s=w402, f="") -> (s? t:f=w399:string)
        n155 = call <vilib>:"Add State(s) to Queue__jki_lib_state_machine.vi"("State(s) in (\"\")"=w399, "State(s) at Back (\"\")"="Data: Cleanup\nExit") -> ("States Out"=w397:string)  [unwired: 13 in]
        n156 = call <vilib>:"Add State(s) to Queue__jki_lib_state_machine.vi"("State(s) in Front (\"\")"=w397, "State(s) in (\"\")"=w406) -> ("States Out"=w405:string)  [unwired: 13 in]
      }
      frame "---------- New Category ----------" {
        # "Template Separator\n(You can make a copy of, or modify, this frame)"
        n157 = call <vilib>:"Add State(s) to Queue__jki_lib_state_machine.vi"("State(s) in (\"\")"=w410) -> ("States Out"=w409:string)  [unwired: 14 in]
      }
      frame "New Category: 1" {
        # "Your code here.\n(You can make a copy of, or modify, this frame)"
        n158 = call <vilib>:"Add State(s) to Queue__jki_lib_state_machine.vi"("State(s) in (\"\")"=w414) -> ("States Out"=w413:string)  [unwired: 14 in]
      }
      frame "New Category: 2" {
        # "Your code here.\n(You can make a copy of, or modify, this frame)"
        n159 = call <vilib>:"Add State(s) to Queue__jki_lib_state_machine.vi"("State(s) in (\"\")"=w418) -> ("States Out"=w417:string)  [unwired: 14 in]
      }
      frame "---------- AWS ----------" {
        # "Template Separator\n(You can make a copy of, or modify, this frame)"
        n160 = call <vilib>:"Add State(s) to Queue__jki_lib_state_machine.vi"("State(s) in (\"\")"=w422) -> ("States Out"=w421:string)  [unwired: 14 in]
      }
      frame "AWS: Initialize" {
        # "need to somehow set credentials and bucket"
        # "Template Separator\n(You can make a copy of, or modify, this frame)"
        n161 = Unbundle By Name(w430) -> ("Data.S3"=w432:refnum<class "Data.S3.lvclass">)
        n162 = call "Read Credentials from File.vi"("error in (no error)"=w424, "path to aws credentials"="path to aws credentials", "Data.S3"=w432) -> ("error out"=w425:errorcluster, "Data.S3 out"=w426:refnum<class "Data.S3.lvclass">)  [unwired: 7 in]
        n163 = call "Set Bucket.vi"("error in (no error)"=w425, "Bucket name"="S3 bucket", "Data.S3"=w426) -> ("error out"=w423:errorcluster, "Data.S3"=w431:refnum<class "Data.S3.lvclass">)  [unwired: 7 in]
        n164 = Bundle By Name(cluster=w430, "Data.S3"=w431) -> (w429:T12)
        n165 = call <vilib>:"Add State(s) to Queue__jki_lib_state_machine.vi"("State(s) in (\"\")"=w434) -> ("States Out"=w433:string)  [unwired: 14 in]
      }
      frame "AWS: Populate Remote Tree" {
        # "Your code here.\n(You can make a copy of, or modify, this frame)"
        n166 = property on="Listing Indicator" class="Bool (strict)"(error in=w440, "Value"=TRUE ("Listing Indicator")) -> (error out=w438:errorcluster)  [unwired: 1 in, 1 out]
        n167 = Unbundle By Name(w448) -> ("Data.S3"=w450:refnum<class "Data.S3.lvclass">)
        n168 = call <userlib>:"Tick Count (ms)__ogtk.vi"("error in (no error)"=w438) -> ("error out"=w442:errorcluster, "millisecond timer value"=w443:u32)  [unwired: 9 in]
        n169 = control-ref of="Remote Tree"() -> (w449:refnum<vi>)
        n170 = call "Populate Tree Ctl from Bucket.vi"("error in (no error)"=w442, "Tree Ctl Ref"=w449, "Data.S3"=w450) -> ("error out"=w441:errorcluster, "Data.S3 out"=w447:refnum<class "Data.S3.lvclass">)  [unwired: 4 in, 3 out]
        n171 = call <userlib>:"Tick Count (ms)__ogtk.vi"("error in (no error)"=w441) -> ("error out"=w436:errorcluster, "millisecond timer value"=w445:u32)  [unwired: 9 in]
        n172 = Subtract(x=w445, y=w443) -> (x-y=→"Remote Tree load (ms)":u32)
        n173 = Bundle By Name(cluster=w448, "Data.S3"=w447) -> (w446:T12)
        n174 = property on="Listing Indicator" class="Bool (strict)"(error in=w436, "Value"=FALSE ("Listing Indicator")) -> (error out=w435:errorcluster)  [unwired: 1 in, 1 out]
        n175 = call <vilib>:"Add State(s) to Queue__jki_lib_state_machine.vi"("State(s) in (\"\")"=w452) -> ("States Out"=w451:string)  [unwired: 14 in]
      }
      frame "AWS: Copy Remote Selection to Local Tree" {
        # "create local folder"
        # "Template Separator\n(You can make a copy of, or modify, this frame)"
        n176 = control-ref of="Local Tree"() -> (w456:refnum<vi>)
        n177 = Unbundle By Name(w467) -> ("Data.S3"=w471:refnum<class "Data.S3.lvclass">, "local bigdata directory"=w470:path, "selected.\\ remote path"=w469:string, "selected./ remote path"=w454:string)
        n178 = property on="Downloading Indicator" class="Bool (strict)"(error in=w462, "Value"=TRUE ("Downloading Indicator")) -> (error out=w457:errorcluster)  [unwired: 1 in, 1 out]
        n179 = call-poly <userlib>:"Build Path__ogtk.vi"("name or relative path"=w469, "base path"=w470) -> ("appended path"=w463:path)
        n180 = call-poly <userlib>:"Strip Path__ogtk.vi"("path"=w463) -> ("stripped path"=w468:path)  [unwired: 1 out]
        n181 = call <userlib>:"Create Dir if Non-Existant__ogtk.vi"("error in (no error)"=w457, "Directory Path"=w468) -> ("error out"=w464:errorcluster)  [unwired: 7 in, 2 out]
        n182 = Path To String(path=w463) -> (string=w455:string)
        n183 = call "recursively populate local tree ctl.vi"("error in (no error)"=w464, "Object path"=w455, "tree ctl ref"=w456) -> ("error out"=w453:errorcluster)  [unwired: 7 in, 1 out]
        n184 = call "Download File.vi"("error in (no error)"=w453, "Object Path"=w454, "path to store downloaded file"=w463, "Data.S3"=w471) -> ("error out"=w459:errorcluster, "Data.S3 out"=w465:refnum<class "Data.S3.lvclass">)  [unwired: 5 in, 1 out]
        n185 = Bundle By Name(cluster=w467, "Data.S3"=w465) -> (w466:T12)
        n186 = property on="Downloading Indicator" class="Bool (strict)"(error in=w459, "Value"=FALSE ("Downloading Indicator")) -> (error out=w458:errorcluster)  [unwired: 1 in, 1 out]
        n187 = call <vilib>:"Add State(s) to Queue__jki_lib_state_machine.vi"("State(s) in (\"\")"=w473) -> ("States Out"=w472:string)  [unwired: 14 in]
      }
      frame "AWS: Upload file" {
        w490 = "/"
        # "SA030.."
        # "031_.."
        # "#TODO: put these values in the\nstate wire..."
        # "Template Separator\n(You can make a copy of, or modify, this frame)"
        n188 = Unbundle By Name(w481) -> ("Data.S3"=w475:refnum<class "Data.S3.lvclass">, "local bigdata directory"=w474:path)
        n189 = Path To String(path=w474) -> (string=w478:string)
        n190 = Concatenate Strings(w478, ".tdms") -> (w493:string)
        n191 = String To Path(string=w493) -> (path=w476:path)
        n192 = Strip Path(path=w476) -> (stripped path=w491:path, name=w488:string)
        n193 = Strip Path(path=w491) -> (name=w486:string)  [unwired: 1 out]
        n194 = call "replace_bad_aws_characters.vi"("error in (no error)"=w484, "name"=w488) -> ("error out"=w483:errorcluster, "result string"=w487:string)  [unwired: 8 in]
        n195 = call "replace_bad_aws_characters.vi"("error in (no error)"=w483, "name"=w486) -> ("error out"=w482:errorcluster, "result string"=w485:string)  [unwired: 8 in]
        n196 = call-poly <userlib>:"File Exists__ogtk.vi"("file path"=w476) -> ("exists"=w492:bool)  [unwired: 6 in, 1 out]
        n197 = Concatenate Strings(w490, w485, w490, w487) -> (w477:string)
        n198 = case shown="False" w492 {
          tunnel: w476 -> [_ w501]
          tunnel: w477 -> [_ w504]
          tunnel: w482 -> [w498 w503]
          tunnel: [w498 w502] -> w489
          tunnel: w475 -> [w497 w500]
          tunnel: [w497 w499] -> w480
          frame False {
            n199 = call "Display Message to User"() -> ()  [unwired: 10 in, 2 out]
          }
          frame True {
            n200 = call "Upload File.vi"("error in (no error)"=w503, "Object Path (including file name)"=w504, "file to upload"=w501, "Data.S3"=w500) -> ("error out"=w502:errorcluster, "Data.S3"=w499:refnum<class "Data.S3.lvclass">)  [unwired: 6 in]
          }
        }
        n201 = Bundle By Name(cluster=w481, "Data.S3"=w480) -> (w479:T12)
        n202 = call <vilib>:"Add State(s) to Queue__jki_lib_state_machine.vi"("State(s) in (\"\")"=w496) -> ("States Out"=w495:string)  [unwired: 14 in]
      }
      frame "AWS: Download file" {
        # "DEPRECATED"
        # "Template Separator\n(You can make a copy of, or modify, this frame)"
        n203 = Unbundle By Name(w505) -> ("Data.S3"=w508:refnum<class "Data.S3.lvclass">, "local bigdata directory"=w506:path)
        n204 = Path To String(path=w506) -> (string=w507:string)
        n205 = call "replace_bad_aws_characters.vi"("error in (no error)"=w510, "name"=w507) -> ("error out"=w509:errorcluster, "result string"=w511:string)  [unwired: 8 in]
        n206 = Concatenate Strings(w511, ".tdms") -> (w514:string)
        n207 = String To Path(string=w514) -> (path=w512:path)
        n208 = call "Download File.vi"("error in (no error)"=w509, "path to store downloaded file"=w512, "Data.S3"=w508) -> ("error out"=w513:errorcluster)  [unwired: 6 in, 2 out]
        n209 = call <vilib>:"Add State(s) to Queue__jki_lib_state_machine.vi"("State(s) in (\"\")"=w517) -> ("States Out"=w516:string)  [unwired: 14 in]
      }
      frame "AWS: Check if file exists" {
        # "DEPRECATED"
        # "Your code here.\n(You can make a copy of, or modify, this frame)"
        n210 = Unbundle By Name(w527) -> ("Data.S3"=w519:refnum<class "Data.S3.lvclass">, "local bigdata directory"=w518:path)
        n211 = Path To String(path=w518) -> (string=w521:string)
        n212 = call "replace_bad_aws_characters.vi"("name"=w521) -> ("result string"=w520:string)  [unwired: 9 in, 1 out]
        n213 = Concatenate Strings(w520, ".tdms") -> (w525:string)
        n214 = String To Path(string=w525) -> (path=w522:path)
        n215 = call "Verify File.vi"("error in (no error)"=w524, "file to check"=w522, "Data.S3"=w519) -> ("error out"=w523:errorcluster)  [unwired: 6 in, 2 out]
        n216 = call <vilib>:"Add State(s) to Queue__jki_lib_state_machine.vi"("State(s) in (\"\")"=w529) -> ("States Out"=w528:string)  [unwired: 14 in]
      }
      frame "---------- PostgreSQL ----------" {
        # "Template Separator\n(You can make a copy of, or modify, this frame)"
        n217 = call <vilib>:"Add State(s) to Queue__jki_lib_state_machine.vi"("State(s) in (\"\")"=w533) -> ("States Out"=w532:string)  [unwired: 14 in]
      }
      frame "PostgreSQL: Configure Connection" {
        # "Template Separator\n(You can make a copy of, or modify, this frame)"
        n218 = Unbundle By Name(w534) -> ("Data.PGSQL"=w539:refnum<class "Data.PGSQL.lvclass">)
        n219 = call <userlib>:"Set Connection Info.vi"("Data.PG in"=w539, "error in (no error)"=w538) -> ("Data.PG out"=w535:refnum<class "Data.PGSQL.lvclass">, "error out"=w537:errorcluster)  [unwired: 7 in]
        n220 = Bundle By Name(cluster=w534, "Data.PGSQL"=w535) -> (w536:T12)
        n221 = call <vilib>:"Add State(s) to Queue__jki_lib_state_machine.vi"("State(s) in (\"\")"=w541) -> ("States Out"=w540:string)  [unwired: 14 in]
      }
      frame "PostgreSQL: Upload Data" {
        # "Template Separator\n(You can make a copy of, or modify, this frame)"
        n222 = call <vilib>:"Add State(s) to Queue__jki_lib_state_machine.vi"("State(s) in (\"\")"=w545) -> ("States Out"=w544:string)  [unwired: 14 in]
      }
      frame "---------- Process ----------" {
        # "Template Separator\n(You can make a copy of, or modify, this frame)"
        n223 = call <vilib>:"Add State(s) to Queue__jki_lib_state_machine.vi"("State(s) in (\"\")"=w549) -> ("States Out"=w548:string)  [unwired: 14 in]
      }
      frame "Process: Slice to XY data" {
        # "#TODO: this should be a typedef?"
        # "#TODO: add ring ctls for channels\n(tdms has a function for this)"
        # "no operations performed\nyet on freshly sliced data"
        # "have 3D array (pages of 2D arrays containing channels vs time)"
        # "Template Separator\n(You can make a copy of, or modify, this frame)"
        n224 = call <userlib>:"Tick Count (ms)__ogtk.vi"("error in (no error)"=w575) -> ("error out"=w564:errorcluster, "millisecond timer value"=w572:u32)  [unwired: 9 in]
        n225 = Unbundle By Name(w571) -> ("Data Save"=w566:refnum<class "Data.lvclass">, "ch selection"=w557:cluster{"X Ch":string, "Y Ch":string}, "data dimensions"=w550:i32[])
        n226 = property on="updating" class="Bool (strict)"(error in=w564, "Value"=TRUE ("updating")) -> ()  [unwired: 1 in, 2 out]
        n227 = call <userlib>:"Read Data (Dictionary).vi"("error in (no error)"=w564, "Data Save"=w566) -> ("error out"=w563:errorcluster, "Data (Dictionary)"=w561:T19[], "Data Save out"=w565:refnum<class "Data.lvclass">)  [unwired: 7 in]
        n228 = call <userlib>:"Read Wavenames.vi"("error in (no error)"=w563, "Data Save"=w565) -> ("error out"=w559:errorcluster, "Wavenames"=→"Wavenames":string[], "Data Save out"=w555:refnum<class "Data.lvclass">)  [unwired: 7 in]
        n229 = Index Array(array=w550) -> (element=w552:i32)  [unwired: 1 in]
        n230 = Unbundle By Name(w557) -> ("X Ch"=w554:string, "Y Ch"=w553:string)
        n231 = call "Data(dictionary) to XY.vi"("dimension size (hmm)"=w552, "chopper params"="chopper params", "error in (no error)"=w559, "IV Y wavename"=w553, "IV X wavename"=w554, "Data (Dictionary)"=w561) -> ("error out"=w558:errorcluster, "wacky arary"=w560:cluster{dbl[], dbl[]}[])  [unwired: 4 in]
        n232 = Bundle By Name(cluster=w571, "Data Save"=w555, "active XY data"=w560, "operations performed"=string[] []) -> (w570:T12)
        n233 = call <userlib>:"Tick Count (ms)__ogtk.vi"("error in (no error)"=w558) -> ("error out"=w574:errorcluster, "millisecond timer value"=w573:u32)  [unwired: 9 in]
        n234 = Subtract(x=w573, y=w572) -> (x-y=→"slicing\ntime":u32)
      }
      frame "Process: Check for Updates" {
        # "if the performed operations\ndon't match the desired list\nthen data needs updated 0_0"
        # "'no need'"
        # "if these are NOT equal\nthen it needs to be resliced\n-> result must be false"
        # "tru if all match"
        # "have 3D array (pages of 2D arrays containing channels vs time)"
        # "Template Separator\n(You can make a copy of, or modify, this frame)"
        n235 = Unbundle By Name(w590) -> ("operations performed"=w576:string[], "Operations List"=w591:refnum<vi>)
        n236 = property on="Property Node" class="LstBox (strict)"(reference=w591) -> ("Item Names"=w577:string[])  [unwired: 1 in, 2 out]
        n237 = Equal?(x=w576, y=w577) -> (x = y?=w579:bool[])
        n238 = And Array Elements(Boolean array=w579) -> (logical AND=w584:bool)
        n239 = Array Size(array=w576) -> (size(s)=w587:i32)
        n240 = Array Size(array=w577) -> (size(s)=w586:i32)
        n241 = Not(x=w584) -> (.not. x?=w578:bool)
        n242 = Not Equal?(x=w587, y=w586) -> (x != y?=w585:bool)
        n243 = Or(x=w578, y=w585) -> (x .or. y?=w583:bool)
        n244 = Select(t="Macro: Reslice and perform all ops", s=w583, f="") -> (s? t:f=w580:string)
        n245 = call <vilib>:"Add State(s) to Queue__jki_lib_state_machine.vi"("State(s) in Front (\"\")"=w580, "State(s) in (\"\")"=w589) -> ("States Out"=w588:string)  [unwired: 13 in]
      }
      frame "Process: Add Operation" {
        # "#OPERATIONS"
        # "have 3D array (pages of 2D arrays containing channels vs time)"
        # "Template Separator\n(You can make a copy of, or modify, this frame)"
        n246 = Unbundle By Name(w600) -> ("dictionary out"=w601:T11)
        n247 = Unbundle By Name(w600) -> ("Operations List"=w599:refnum<vi>)
        n248 = case shown="\"fft\"" "Operation Config" {
          tunnel: [w605 w611] -> w604
          tunnel: w601 -> [w608 w613]
          tunnel: w603 -> [w607 w615]
          tunnel: [w606 w614] -> w602
          frame "derivative", Default {
            # "key = stringified derivative\nvalue = the derivative parameter cluster"
            n249 = call "derivative_toString.vi"("derivative"="derivative") -> ("concatenated string"=w605:string)  [unwired: 10 in]
            n250 = Bundle("concatenated string"=w605, "derivative"="derivative") -> (w610:T20)  [unwired: 1 in]
            n251 = call-poly <userlib>:"Dictionary Update__ogtk.vi"("error in (no error)"=w607, "key-value"=w610, "dictionary"=w608) -> ("error out"=w606:errorcluster)  [unwired: 6 in, 2 out]
          }
          frame "fft" {
            w611 = "fft"
            n252 = Bundle(w611, "fft"=T9 {"fft"="fft"}) -> (w616:cluster{string, "fft":T9})  [unwired: 1 in]
            n253 = call-poly <userlib>:"Dictionary Update__ogtk.vi"("error in (no error)"=w615, "key-value"=w616, "dictionary"=w613) -> ("error out"=w614:errorcluster)  [unwired: 6 in, 2 out]
          }
        }
        n254 = property on="Property Node" class="LstBox (strict)"(reference=w599) -> (reference out=w596:refnum<vi>, "Item Names"=w598:string[])  [unwired: 1 in, 1 out]
        n255 = Build Array (concatenate)(w598, w604) -> (w597:string[])
        n256 = property on="Property Node" class="LstBox (strict)"(reference=w596, "Item Names"=w597, "Val(Sgnl)"=0 ("Value (Signaling)")) -> ()  [unwired: 1 in, 2 out]
      }
      frame "Process: Perform All Operations" {
        # "dict keys are \nunique operation \nidentifier strings"
        # "have 3D array (pages of 2D arrays containing channels vs time)"
        # "Template Separator\n(You can make a copy of, or modify, this frame)"
        n257 = Unbundle By Name(w623) -> ("dictionary out"=w619:T11, "Operations List"=w625:refnum<vi>)
        n258 = property on="Property Node" class="LstBox (strict)"(reference=w625) -> ("Item Names"=w617:string[])  [unwired: 1 in, 2 out]
        n259 = Unbundle By Name(w623) -> ("active XY data"=w621:T17)
        n260 = for {
          tunnel: w617 -> [w637] mode=indexing
          shift-right: [w636] -> _
          shift-left: w619 -> [w626]
          shift-right: [w628] -> _
          shift-left: _ -> [w633]
          shift-right: [w630] -> w618
          shift-left: w621 -> [w631]
          tunnel: [w627] -> _ mode=indexing
          # "the label of the first cluster element must describe the operation"
          # "#OPERATIONS"
          n261 = call <userlib>:"Dictionary Get Value__ogtk.vi"("error in"=w633, "key"=w637, "dictionary"=w626) -> ("error out"=w634:errorcluster, "value"=w632:variant, "dictionary out"=w636:T11)  [unwired: 5 in, 1 out]
          n262 = call <userlib>:"Get Cluster Element Names__ogtk.vi"("error in (no error)"=w634, "Cluster"=w632) -> ("error out"=w629:errorcluster, "Element Names"=w635:string[])  [unwired: 8 in]
          n263 = Index Array(array=w635) -> (element=w627:string)  [unwired: 1 in]
          n264 = case shown="\"derivative\"" w627 {
            tunnel: w632 -> [_ w652]
            tunnel: w631 -> [w643 w650]
            tunnel: [w639 w649] -> w630
            tunnel: w629 -> [w642 w651]
            tunnel: [w640 w648] -> w628
            frame "fft", Default {
              n265 = call <userlib>:"FFT (multiple).vi"("error in (no error)"=w642, "XY-data"=w643) -> ("error out"=w641:errorcluster, "magnitude []"=w638:cluster{"f0":dbl, "df":dbl, "magnitude":dbl[]}[])  [unwired: 6 in, 2 out]
              n266 = call "freq_magnitude_to_XY.vi"("error in (no error)"=w641, "magnitude []"=w638) -> ("error out"=w640:errorcluster, "freq_magnitude_XY"=w639:cluster{dbl[], "magnitude":dbl[]}[])  [unwired: 8 in]
            }
            frame "derivative" {
              n267 = Variant To Data(type=T10 {"derivative"="derivative", "Interval"=2.0, "Interval Units"=enum."Points", "Type"=enum."dy/dx vs x"} ("derivative"), Variant=w652) -> (data=w653:T10)  [unwired: 1 in, 1 out]
              n268 = Unbundle By Name(w653) -> ("Interval"=w647:dbl, "Interval Units"=w645:enum16{"Points", "Data"}, "Type"=w646:enum16{"dy/dx vs x", "dx/dy vs y"})
              n269 = call-poly <userlib>:"Derivative.vi"("Interval Units"=w645, "error in (no error)"=w651, "Type"=w646, "Interval"=w647, "XY-data"=w650) -> ("error out"=w648:errorcluster, "Differential out"=w649:cluster{"X-array":dbl[], "Y-array":dbl[]}[])  [unwired: 4 in, 1 out]
            }
          }
        }
        n270 = Bundle By Name(cluster=w623, "active XY data"=w618, "operations performed"=w617) -> (w622:T12)
      }
      frame "---------- Visualize ----------" {
        # "Template Separator\n(You can make a copy of, or modify, this frame)"
        n271 = call <vilib>:"Add State(s) to Queue__jki_lib_state_machine.vi"("State(s) in (\"\")"=w657) -> ("States Out"=w656:string)  [unwired: 14 in]
      }
      frame "Visualize: Plot Live XY to Intensity" {
        # "?"
        # "?"
        # "#TODO: only supports 1st scan for now"
        # "#TODO: Shouldnt go in here"
        n272 = control-ref of="Intensity Graph"() -> (w679:refnum<vi>)
        n273 = Unbundle By Name(w658) -> ("scan info"=w687:T14, "graphs"=w700:refnum<class "graph_utilities.lvclass">[], "active XY data"=w699:T17)
        n274 = property class="IntGraph (strict)"(reference=w679, error in=w678, "XScale.ScaleFit"=u8 0 ("X Scale.Scale Fit")) -> (reference out=w674:refnum<vi>, error out=w677:errorcluster)
        n275 = Unbundle By Name(w687) -> ("scan names"=w686:string[], "starts"=w683:dbl[], "ends"=w684:dbl[], "steps"=w685:dbl[])
        n276 = call "XYs_to_Intensity.vi"("error in (no error)"=w677, "XYs in"=w699) -> ("error out"=w698:errorcluster, "Intensity data (y) out"=w667:dbl[][])  [unwired: 8 in]
        n277 = Index Array(array=w700) -> (element=w701:refnum<class "graph_utilities.lvclass">)  [unwired: 1 in]
        n278 = Array Size(array=w667) -> (size(s)=w666:i32[])
        n279 = call <userlib>:"Set Intensity Graph Value.vi"("error in (no error)"=w698, "Value"=w667, "graph_utilities in"=w701) -> ("error out"=w693:errorcluster, "graph_utilities out"=w694:refnum<class "graph_utilities.lvclass">)  [unwired: 7 in]
        n280 = Index Array(array=w666) -> (element #1=w665:i32)  [unwired: 3 in, 2 out]
        n281 = Index Array(array=w684) -> (element=w663:dbl)  [unwired: 1 in]
        "intended sweep end" <- w663
        n282 = Index Array(array=w686) -> (element=w682:string)  [unwired: 1 in]
        n283 = Index Array(array=w683) -> (element=w660:dbl)  [unwired: 1 in]
        n284 = Index Array(array=w685) -> (element=w668:dbl)  [unwired: 1 in]
        n285 = call <userlib>:"Set Intensity Graph Z Color.vi"("error in (no error)"=w693, "Colors []"=u32[] [10420479, 16860, 3381759, 6618880, 16772608, 16711680], "graph_utilities in"=w694) -> ("error out"=w671:errorcluster, "graph_utilities out"=w672:refnum<class "graph_utilities.lvclass">)  [unwired: 7 in]
        n286 = Multiply(x=w668, y=w665) -> (x*y=w664:dbl)
        n287 = Add(x=w660, y=w664) -> (x+y=w662:dbl)
        "actual sweep end" <- w662
        n288 = Select(t=w663, s="intended (t) end\nactual (f) end", f=w662) -> (s? t:f=w659:dbl)
        n289 = call <userlib>:"Set Intensity Graph X Scale Min and Max.vi"("error in (no error)"=w671, "End [1]"=w659, "Start [0]"=w660, "graph_utilities in"=w672) -> ("error out"=w669:errorcluster, "graph_utilities out"=w670:refnum<class "graph_utilities.lvclass">)  [unwired: 6 in]
        n290 = call <userlib>:"Set Intensity Graph X Label.vi"("error in (no error)"=w669, "X Label"=w682, "graph_utilities in"=w670) -> ("error out"=w691:errorcluster, "graph_utilities out"=w689:refnum<class "graph_utilities.lvclass">)  [unwired: 7 in]
        n291 = call <userlib>:"Set Intensity Graph Y Label.vi"("error in (no error)"=w691, "Y Label"="Entire IV", "graph_utilities in"=w689) -> ("error out"=w690:errorcluster, "graph_utilities out"=w688:refnum<class "graph_utilities.lvclass">)  [unwired: 7 in]
        n292 = call <userlib>:"Set Intensity Graph Z Label.vi"("error in (no error)"=w690, "graph_utilities in"=w688) -> ("error out"=w675:errorcluster)  [unwired: 8 in, 1 out]
        n293 = property class="IntGraph (strict)"(reference=w674, error in=w675, "XScale.ScaleFit"=u8 1 ("X Scale.Scale Fit")) -> (error out=w676:errorcluster)  [unwired: 1 out]
        n294 = property on="updating" class="Bool (strict)"(error in=w676, "Value"=FALSE ("updating")) -> (error out=w697:errorcluster)  [unwired: 1 in, 1 out]
        n295 = call <vilib>:"Add State(s) to Queue__jki_lib_state_machine.vi"("State(s) in Front (\"\")"="Visualize: Calculate Histogram" ("State(s) in Front (\"\")"), "State(s) in (\"\")"=w703) -> ("States Out"=w702:string)  [unwired: 13 in]
      }
      frame "Visualize: Calculate Histogram" {
        n296 = Unbundle By Name(w708) -> ("graphs"=w707:refnum<class "graph_utilities.lvclass">[])
        n297 = Index Array(array=w707) -> (element=w706:refnum<class "graph_utilities.lvclass">)  [unwired: 1 in]
        n298 = disable-structure shown="Enabled" {
          disable-tunnel: w706 -> [_ w727]
          disable-tunnel: w710 -> [w722 w726]
          disable-tunnel: [w715 w725] -> w709
          disable-tunnel: "# std deviations for histogram width" -> [w713 w724]
          disable-tunnel: "lock to bin edges" -> [_ w723]
          frame Disabled {
            n299 = call "XYs_to_Intensity.vi"("error in (no error)"=w722) -> ("error out"=w720:errorcluster, "Intensity data (y) out"=w721:dbl[][])  [unwired: 9 in]
            n300 = call "calculate_histogram.vi"("error in (no error)"=w720, "# std deviations for histogram width (1)"=w713, "2D arr Intensity Graph"=w721) -> ("error out"=w718:errorcluster, "Histogram Graph"=w719:T16)  [unwired: 5 in, 2 out]
            n301 = property class="XYGraph (strict)"(error in=w718, "Value"=w719) -> (reference out=w717:refnum<vi>, error out=w716:errorcluster)  [unwired: 1 in]
            n302 = call "adjust_histogram_cursor.vi"("error in (no error)"=w716, "lock to bin edges"=TRUE, "histogram reference"=w717) -> ("error out"=w715:errorcluster)  [unwired: 8 in]
          }
          frame Enabled {
            n303 = call <userlib>:"Intensity Graph Histogram Control.vi"("error in (no error)"=w726, "lock to bin edges"=w723, "# std deviations for histogram width"=w724, "graph_utilities in"=w727) -> ("error out"=w725:errorcluster)  [unwired: 4 in, 3 out]
          }
        }
        n304 = call <vilib>:"Add State(s) to Queue__jki_lib_state_machine.vi"("State(s) in (\"\")"=w712) -> ("States Out"=w711:string)  [unwired: 14 in]
      }
      frame "Visualize: Update Z from Histogram" {
        n305 = disable-structure shown="Disabled" {
          disable-tunnel: w730 -> [w747 w756 _]
          disable-tunnel: w729 -> [w742 w754 w763]
          disable-tunnel: [w741 w750 w763] -> w728
          frame Disabled {
            # "#TODO: adjust line cut scales\nhere also"
            n306 = Unbundle By Name(w747) -> ("graphs"=w744:refnum<class "graph_utilities.lvclass">[])  [unwired: 1 out]
            n307 = property on="Property Node" class="XYGraph (strict)"(error in=w742, "Active Cursor"=u32 0, "Active Cursor"=u32 1) -> (error out=w737:errorcluster, "Cursor.Cursor X"=w736:dbl, "Cursor.Cursor X"=w735:dbl)  [unwired: 1 in, 1 out]
            n308 = control-ref of="Horizontal Linecut"() -> (w734:refnum<vi>)
            n309 = control-ref of="Vertical Linecut"() -> (w733:refnum<vi>)
            n310 = disable-structure shown="Enabled" {
              disable-tunnel: w744 -> [w748 _]
              disable-tunnel: [_ w749] -> w743
              frame Disabled {
                # "Should have a graphutils\nvi for Z range setting here"
                n311 = Index Array(array=w748) -> ()  [unwired: 1 in, 1 out]
              }
              frame Enabled {
                n312 = control-ref of="Intensity Graph"() -> (w749:refnum<vi>)
              }
            }
            n313 = property on="Property Node" class="IntGraph (strict)"(reference=w743, error in=w737, "ZScale.Minimum"=w736, "ZScale.Maximum"=w735) -> (error out=w740:errorcluster)  [unwired: 1 out]
            n314 = property on="Property Node" class="XYGraph (strict)"(reference=w734, error in=w737, "YScale.Minimum"=w736, "YScale.Maximum"=w735) -> (error out=w739:errorcluster)  [unwired: 1 out]
            n315 = property on="Property Node" class="XYGraph (strict)"(reference=w733, error in=w737, "YScale.Minimum"=w736, "YScale.Maximum"=w735) -> (error out=w738:errorcluster)  [unwired: 1 out]
            n316 = Merge Errors(w740, w739, w738) -> (w741:errorcluster)
          }
          frame Disabled {
            # "This is taken care of by Intensity Graph Histogram Control.vi"
            n317 = Unbundle By Name(w756) -> ("graphs"=w757:refnum<class "graph_utilities.lvclass">[])
            n318 = Index Array(array=w757) -> (element=w755:refnum<class "graph_utilities.lvclass">)  [unwired: 1 in]
            n319 = call <userlib>:"Read XY Graph ref.vi"("error in (no error)"=w754, "graph_utilities in"=w755) -> ("error out"=w751:errorcluster, "XY Graph"=w752:refnum<vi>, "graph_utilities out"=w753:refnum<class "graph_utilities.lvclass">)  [unwired: 6 in, 1 out]
            n320 = property on="Property Node" class="XYGraph"(reference=w752, error in=w751, "Active Cursor"=u32 0, "Active Cursor"=u32 1) -> (error out=w760:errorcluster, "Cursor.Cursor X"=w759:dbl, "Cursor.Cursor X"=w758:dbl)  [unwired: 1 out]
            n321 = call <userlib>:"Set Intensity Graph Z Range.vi"("error in (no error)"=w760, "Maximum [1]"=w758, "Minimum [0]"=w759, "graph_utilities in"=w753) -> ("error out"=w750:errorcluster)  [unwired: 6 in, 1 out]
          }
          frame Enabled {
          }
        }
        n322 = call <vilib>:"Add State(s) to Queue__jki_lib_state_machine.vi"("State(s) in (\"\")"=w732) -> ("States Out"=w731:string)  [unwired: 14 in]
      }
      frame "Visualize: Line Cuts" {
        n323 = disable-structure shown="Disabled" {
          frame Disabled {
            n324 = call <userlib>:"Linecut Example.vi"() -> ()  [unwired: 12 in]
          }
          frame Enabled {
          }
        }
        n325 = Unbundle By Name(w765) -> ("graphs"=w771:refnum<class "graph_utilities.lvclass">[])
        n326 = Index Array(array=w771, index #1=1 ("index"), index #2=2 ("index")) -> (element #1=w770:refnum<class "graph_utilities.lvclass">, element #2=w769:refnum<class "graph_utilities.lvclass">)
        n327 = call <userlib>:"Intensity Graph Linecut (Vertical).vi"("error in (no error)"=w767, "graph_utilities in"=w770) -> ("error out"=w768:errorcluster)  [unwired: 8 in, 1 out]
        n328 = call <userlib>:"Intensity Graph Linecut (Horizontal).vi"("error in (no error)"=w768, "graph_utilities in"=w769) -> ("error out"=w766:errorcluster)  [unwired: 8 in, 1 out]
        n329 = call <vilib>:"Add State(s) to Queue__jki_lib_state_machine.vi"("State(s) in (\"\")"=w774) -> ("States Out"=w773:string)  [unwired: 14 in]
      }
      frame "---------- Load ----------" {
        # "Template Separator\n(You can make a copy of, or modify, this frame)"
        n330 = call <vilib>:"Add State(s) to Queue__jki_lib_state_machine.vi"("State(s) in (\"\")"=w778) -> ("States Out"=w777:string)  [unwired: 14 in]
      }
      frame "Load: Populate Local Tree" {
        # "only show tdms files"
        n331 = Unbundle By Name(w789) -> ("local bigdata directory"=w780:path)
        n332 = call <vilib>:"Recursive File List.vi"("pattern"="*.tdms" ("y"), "error in (no error)"=w783, "Folder Path"=w780) -> ("error out"=w784:errorcluster, "All Files in Dir"=w785:path[])  [unwired: 4 in, 3 out]
        n333 = control-ref of="Local Tree"() -> (w782:refnum<vi>)
        n334 = invoke class="Tree (strict)" method="Edit Tree Items.Delete"(reference=w782, error in=w784) -> (reference out=w788:refnum<vi>, error out=w786:errorcluster)  [unwired: 3 in, 3 out]
        n335 = Path To String(path=w785) -> (string=w781:string[])
        n336 = for {
          tunnel: w788 -> [w792]
          tunnel: w781 -> [w793] mode=indexing
          shift-right: [w794] -> w787
          shift-left: w786 -> [w795]
          n337 = call "recursively populate local tree ctl.vi"("error in (no error)"=w795, "Object path"=w793, "tree ctl ref"=w792) -> ("error out"=w794:errorcluster)  [unwired: 7 in, 1 out]
        }
        n338 = call <vilib>:"Add State(s) to Queue__jki_lib_state_machine.vi"("State(s) in (\"\")"=w791) -> ("States Out"=w790:string)  [unwired: 14 in]
      }
      frame "Load: Load Selected File" {
        # "#TODO: clean up frame with more subvis\nalso this will get messed up if a 'single data\npoint' channel is the first one..."
        # "Template Separator\n(You can make a copy of, or modify, this frame)"
        n339 = Unbundle By Name(w817) -> ("Data Save"=w811:refnum<class "Data.lvclass">, "selected.local path"=w797:path)
        n340 = property on="Loading Indicator" class="Bool (strict)"(error in=w821, "Value"=TRUE ("read cache")) -> (error out=w813:errorcluster)  [unwired: 1 in, 1 out]
        n341 = call <userlib>:"Tick Count (ms)__ogtk.vi"("error in (no error)"=w813) -> ("error out"=w802:errorcluster, "millisecond timer value"=w796:u32)  [unwired: 9 in]
        n342 = call <userlib>:"Data Read.vi"("Append Index"=-1, "error in (no error)"=w802, "path"=w797) -> ("error out"=w810:errorcluster, "Notes"=→"Notes":string, "Data (Dictionary)"=w799:T19[])  [unwired: 5 in, 1 out]
        n343 = call <userlib>:"Write Data (Dictionary).vi"("error in (no error)"=w810, "Data (Dictionary)"=w799, "Data Save"=w811) -> ("error out"=w808:errorcluster, "Data Save out"=w809:refnum<class "Data.lvclass">)  [unwired: 7 in]
        n344 = call <userlib>:"Read Wavenames.vi"("error in (no error)"=w808, "Data Save"=w809) -> ("error out"=w803:errorcluster, "Wavenames"=w800:string[], "Data Save out"=w801:refnum<class "Data.lvclass">)  [unwired: 7 in]
        n345 = call "TDMS Get Number of Groups.vi"("error in (no error)"=w803, "path"=w797) -> ("error out"=w805:errorcluster, "# of groups"=w806:i32)  [unwired: 8 in]
        n346 = call "get data dimensions.vi"("# of groups"=w806, "Data (Dictionary)"=w799) -> ("data dimensions"=w798:i32[])  [unwired: 8 in, 1 out]
        "data dimensions" <- w798
        n347 = call <userlib>:"Tick Count (ms)__ogtk.vi"("error in (no error)"=w805) -> ("error out"=w812:errorcluster, "millisecond timer value"=w815:u32)  [unwired: 9 in]
        n348 = Subtract(x=w815, y=w796) -> (x-y=→"TDMS load (ms)":u32)
        n349 = Bundle By Name(cluster=w817, "Data Save"=w801, "wavenames"=w800, "data dimensions"=w798) -> (w816:T12)
        n350 = property on="Loading Indicator" class="Bool (strict)"(error in=w812, "Value"=FALSE ("read cache")) -> (error out=w819:errorcluster)  [unwired: 1 in, 1 out]
        n351 = call <vilib>:"Add State(s) to Queue__jki_lib_state_machine.vi"("State(s) in (\"\")"=w823) -> ("States Out"=w822:string)  [unwired: 14 in]
      }
      frame "Load: Load Metadata" {
        # "#TODO: clean up frame with more subvis\nalso this will get messed up if a 'single data\npoint' channel is the first one..."
        # "Template Separator\n(You can make a copy of, or modify, this frame)"
        n352 = Unbundle By Name(w837) -> ("channel selection trees"=w834:T13, "selected.local path"=w825:path)
        n353 = call "Read Metadata from TDMS.vi"("error in (no error)"=w835, "file path"=w825) -> ("error out"=w828:errorcluster, "wiring config"=w831:string[][], "scan info"=w824:T5)  [unwired: 7 in]
        "scan info" <- w824
        "wiring config" <- w831
        n354 = Unbundle By Name(w834) -> ("X Scale Selection"=w833:refnum<vi>, "Y Scale Selection"=w832:refnum<vi>)
        n355 = call "populate_channel_tree.vi"("error in (no error)"=w828, "AI or AO"="AO", "wiring config"=w831, "reference"=w833) -> ("error out"=w827:errorcluster)  [unwired: 6 in, 1 out]
        n356 = call "populate_channel_tree.vi"("error in (no error)"=w827, "AI or AO"="AI", "wiring config"=w831, "reference"=w832) -> ("error out"=w826:errorcluster)  [unwired: 6 in, 1 out]
        n357 = Bundle By Name(cluster=w837, "scan info"=w824, "wiring config"=w831) -> (w836:T12)
        n358 = call <vilib>:"Add State(s) to Queue__jki_lib_state_machine.vi"("State(s) in (\"\")"=w839) -> ("States Out"=w838:string)  [unwired: 14 in]
      }
    }
  }
